vi "NAO_UTILIZAR_para_desenvolver.vi"() -> ()   [LabVIEW 2020]
uses:
  <vilib>/Rock Robotics/WPI/RobotDrive/WPI_RobotDriveArcadeDrive_Standard(NoSaturation).vi
  <vilib>/Rock Robotics/Network Tables/NT Read Number.vi
  Prog_Testes/GlobalVariables.vi
  <vilib>/Rock Robotics/Network Tables/NT Write Number.vi
  <vilib>/Rock Robotics/WPI/ThirdParty/Phoenix-LabVIEW/Motor Controller/Controls/CTRE_Phoenix_MotorControl_ControlMode.ctl
  <vilib>/functionblocks/FB Core/FB Core.xnode
  <vilib>/functionblocks/Control/PID/PID.vi
  <vilib>/functionblocks/NI_FunctionBlock Libraries.lvlib
  <vilib>/Rock Robotics/SystemInterfaces/DIO/FPGA_DIOPWMChannel.ctl
  <vilib>/Rock Robotics/WPI/PWM/WPI_PWMDeadband.ctl
  <vilib>/Rock Robotics/WPI/MotorControl/WPI_MotorControlType.ctl
  <vilib>/Rock Robotics/SystemInterfaces/DIO/FPGA_DIOChannel.ctl
  <vilib>/Rock Robotics/WPI/MotorControl/WPI_MotorControlDeviceRef.ctl
  <vilib>/Rock Robotics/WPI/RobotDrive/WPI_RobotDriveDevRef.ctl
panel:
  out "Distance":dbl
  in  "Stop_PID":bool=TRUE
  out "pidOut":dbl
  out "Stop_pid":bool=TRUE
  out "Stop_pid":bool=TRUE
  out "OUT_PUT 2":bool
  out "pwm_shot 2":dbl
  out "Disp_Valido 2":dbl
  out "Axes[1] 2":dbl
  out "Axes[2] 2":dbl
  out "Axes[3] 2":dbl
  in  "input cluster 2":T1
  out "L_Y 2":dbl
  out "L_X 2":dbl
  out "Motor Values  2":dbl[](array[numeric])
  out "RobotDriveDevRef 2":T2={"DevStatus"={"status"=FALSE, "code"=0, "source"=""}, "Motors[]"=[], "Square Inputs"=FALSE, "Max Output"=1.0}
  in  "x 2":dbl
  out "x+y 2":dbl
  in  "Mot_Min 2":dbl=0.35
  in  "Mot_Max 2":dbl=0.35
  out "Lime_Max 2":dbl=0.35
  out "Lime_Min 2":dbl=0.35
  out "Negar 2":bool
  out "output cluster 2":T8
  out "Multiplicação 6":dbl
  out "Buttons 15":bool
  out "Buttons 14":bool
  out "OUT 6":dbl
  out "Mutliple":dbl
  out "Buttons 13":bool
  out "Buttons 12":bool
  out "OUT 5":dbl
  out "Mutliple":dbl
  out "Buttons 11":bool
  out "Buttons 10":bool
  out "OUT 4":dbl
  out "OUT 3":dbl
  out "Buttons 9":bool
  out "Buttons 8":bool
  out "Multiplicação 3":dbl
  out "OUT_PUT":bool
  out "Disp_Valido":dbl
  out "pwm_shot":dbl
  out "Negar":bool
  out "Lime_Min":dbl=0.35
  out "Lime_Max":dbl=0.35
  in  "Mot_Max":dbl=0.35
  in  "Mot_Min":dbl=0.35
  out "x+y":dbl
  in  "x":dbl
  out "RobotDriveDevRef":T2={"DevStatus"={"status"=FALSE, "code"=0, "source"=""}, "Motors[]"=[], "Square Inputs"=FALSE, "Max Output"=1.0}
  out "Motor Values":dbl[](array[numeric])
  out "L_Y":dbl
  out "L_X":dbl
  in  "input cluster":T1
  out "Axes[3]":dbl
  out "Axes[2]":dbl
  out "Axes[1]":dbl
  out "output cluster":T8
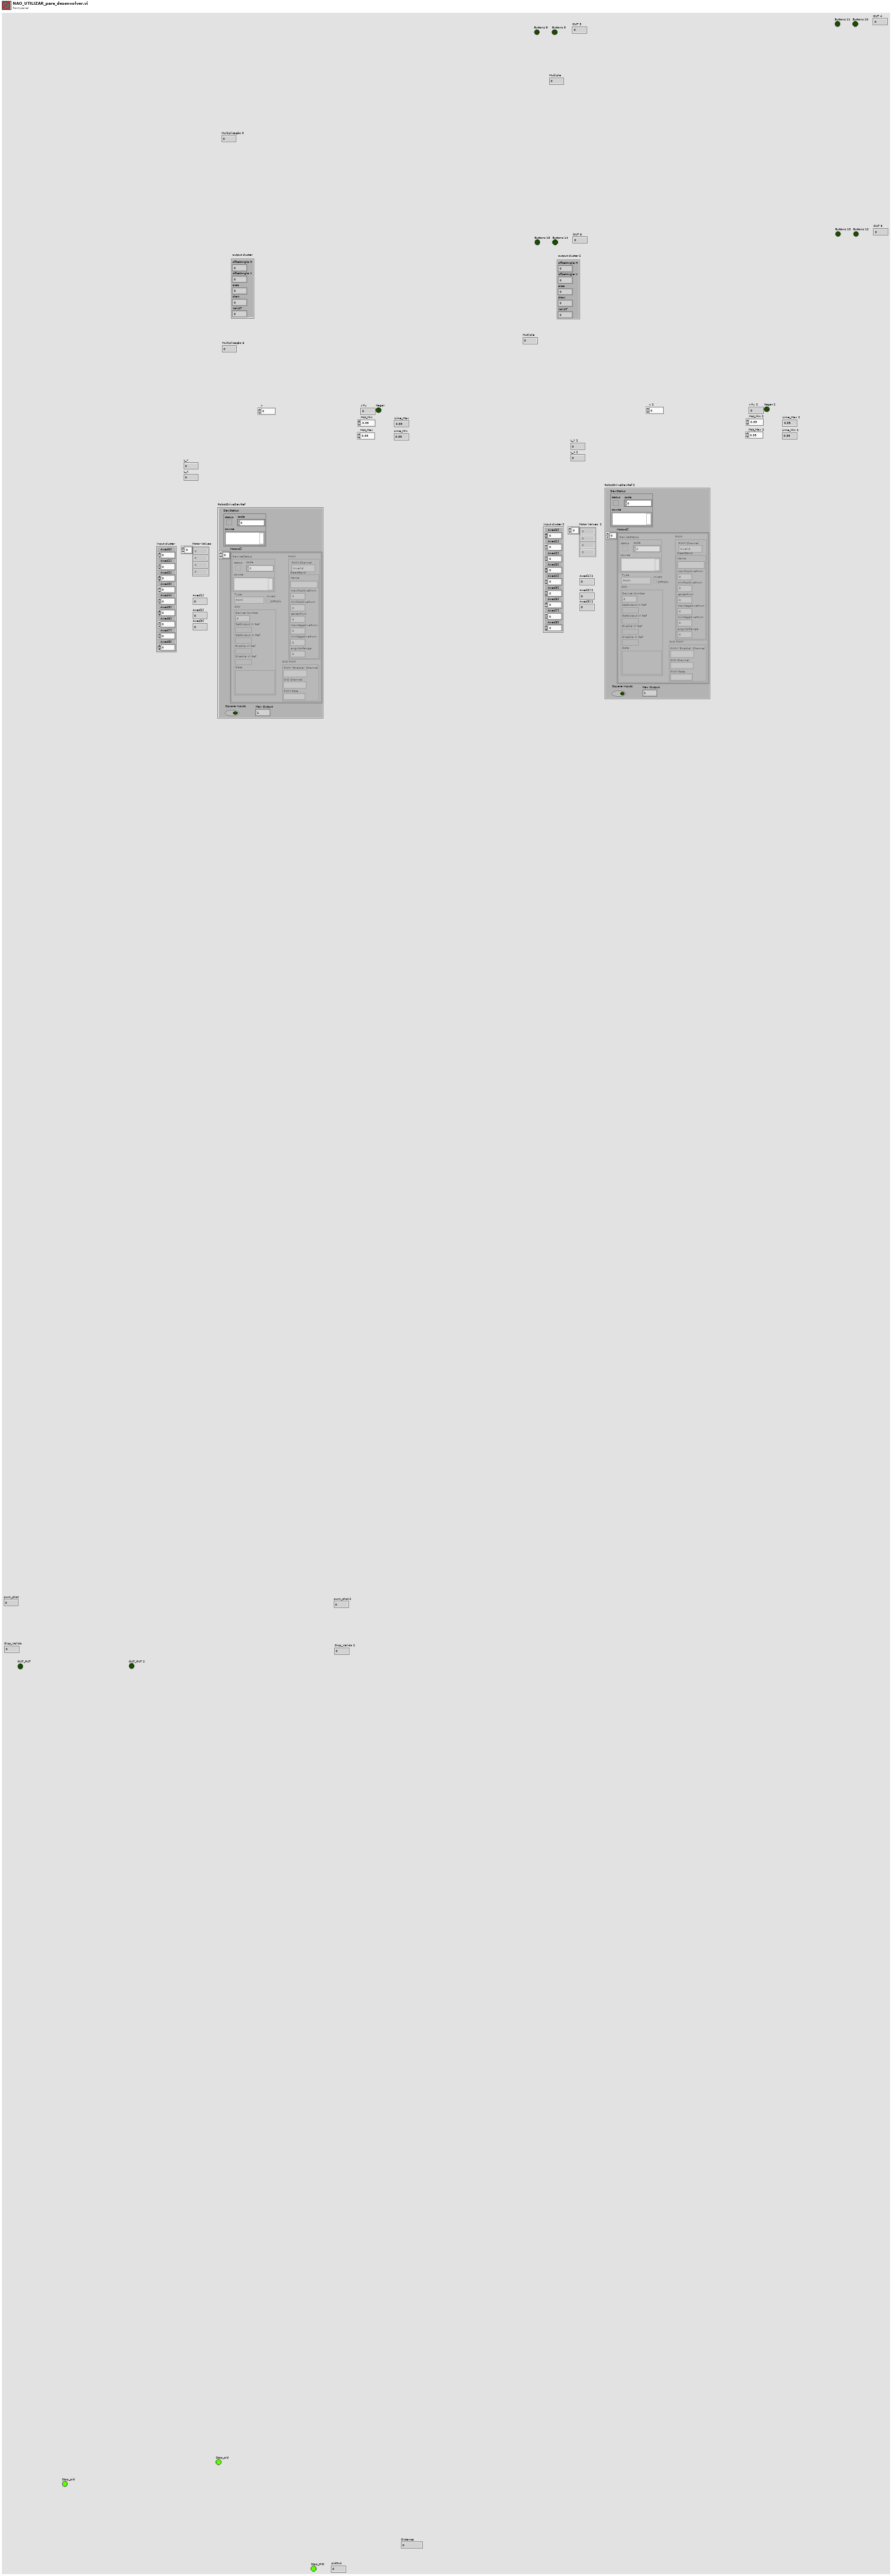
[diagram p1: front panel]
types:
  T1 = cluster{"Axes[0]":dbl, "Axes[1]":dbl, "Axes[2]":dbl, "Axes[3]":dbl, "Axes[4]":dbl, "Axes[5]":dbl, "Axes[6]":dbl, "Axes[7]":dbl, "Axes[8]":dbl}
  T2 = typedef "WPI_RobotDriveDevRef.ctl" = cluster{"DevStatus":errorcluster, "Motors[]":T3[], "Square Inputs":bool, "Max Output":dbl}
  T3 = typedef "WPI_MotorControlDeviceRef.ctl" = cluster{"DeviceStatus":errorcluster, "Type":T4, "PWM":cluster{"PWM Channel":T5, "DeadBand":T6}, "CAN":cluster{"Device Number":u8, "SetOutput VI Ref":variant, "GetOutput VI Ref":variant, "Enable VI Ref":variant, "Disable VI Ref":variant, "Data":variant}, "Invert":bool, "DIO PWM":cluster{"PWM \"Enable\" Channel":T5, "DIOChannel":T7, "PWM Rate":dbl}}
  T4 = typedef "WPI_MotorControlType.ctl" = enum16{"PWM", "CAN", "DIO PWM"}
  T5 = typedef "FPGA_DIOPWMChannel.ctl" = enum8{"PWM 0", "PWM 1", "PWM 2", "PWM 3", "PWM 4", "PWM 5", "PWM 6", "PWM 7", "PWM 8", "PWM 9", "PWM MXP 0", "PWM MXP 1", "PWM MXP 2", "PWM MXP 3", "PWM MXP 4", "PWM MXP 5", "PWM MXP 6", "PWM MXP 7", "PWM MXP 8", "PWM MXP 9", "Invalid"}
  T6 = typedef "WPI_PWMDeadband.ctl" = cluster{"Name":string, "maxPositivePwm":i32, "minPositivePwm":i32, "centerPwm":i32, "maxNegativePwm":i32, "minNegativePwm":i32, "angularRange":u16}
  T7 = typedef "FPGA_DIOChannel.ctl" = enum8{"DIO 0", "DIO 1", "DIO 2", "DIO 3", "DIO 4", "DIO 5", "DIO 6", "DIO 7", "DIO 8", "DIO 9", "DIO MXP 0", "DIO MXP 1", "DIO MXP 2", "DIO MXP 3", "DIO MXP 4", "DIO MXP 5", "DIO MXP 6", "DIO MXP 7", "DIO MXP 8", "DIO MXP 9", "DIO MXP 10", "DIO MXP 11", "DIO MXP 12", "DIO MXP 13", "DIO MXP 14", "DIO MXP 15", "SPI Port CS1", "SPI Port CS2", "SPI Port CS3", "SPI Port MISO", "SPI Port MOSI", "Invalid"}
  T8 = cluster{"offsetAngle H":dbl, "offsetAngle V":dbl, "area":dbl, "skew":dbl, "ValidT":dbl}
  T9 = typedef "CTRE_Phoenix_MotorControl_ControlMode.ctl" = u16
  T10 = cluster{"Buttons[0]":bool, "Buttons[1]":bool, "Buttons[2]":bool, "Buttons[3]":bool, "Buttons[4]":bool, "Buttons[5]":bool, "Buttons[6]":bool, "Buttons[7]":bool, "Buttons[8]":bool, "Buttons[9]":bool}
  T11 = typedef "WPI_JoystickDevRef.ctl" = cluster{"Device":T12}
  T12 = typedef "WPI_JoystickDeviceEnum.ctl" = enum16{"USB 0", "USB 1", "USB 2", "USB 3", "USB 4", "USB 5"}
  T13 = cluster{"Buttons[0]":bool, "Buttons[1]":bool, "Buttons[2]":bool, "Buttons[3]":bool, "Buttons[4]":bool, "Buttons[5]":bool, "Buttons[6]":bool, "Buttons[7]":bool, "Buttons[8]":bool}
  T14 = cluster{"POVs[0]":i16, "POVs[1]":i16, "POVs[2]":i16, "POVs[3]":i16, "POVs[4]":i16, "POVs[5]":i16, "POVs[6]":i16, "POVs[7]":i16}
  T15 = typedef "WPI_EncoderDevRef.ctl" = cluster{"DevStatus":errorcluster, "EncoderIndex":T16, "CounterIndex":T17, "DistancePerCount":dbl, "Decoding Type":T18}
  T16 = typedef "FPGA_EncoderIdx.ctl" = enum8{"Enc 0", "Enc 1", "Enc 2", "Enc 3", "Enc 4", "Enc 5", "Enc 6", "Enc 7", "Invalid"}
  T17 = typedef "FPGA_CounterCtrSystemIndex.ctl" = enum8{"Ctr 0", "Ctr 1", "Ctr 2", "Ctr 3", "Ctr 4", "Ctr 5", "Ctr 6", "Ctr 7", "Invalid"}
  T18 = typedef "WPI_EncoderType.ctl" = enum16{"1x", "2x", "4x"}
  T19 = cluster{"Axes[0]":dbl, "Axes[1]":dbl, "Axes[2]":dbl, "Axes[3]":dbl}
  T20 = cluster{"Axes[0]":dbl, "Axes[1]":dbl, "Axes[2]":dbl, "Axes[3]":dbl, "Axes[4]":dbl, "Axes[5]":dbl, "Axes[6]":dbl, "Axes[7]":dbl}
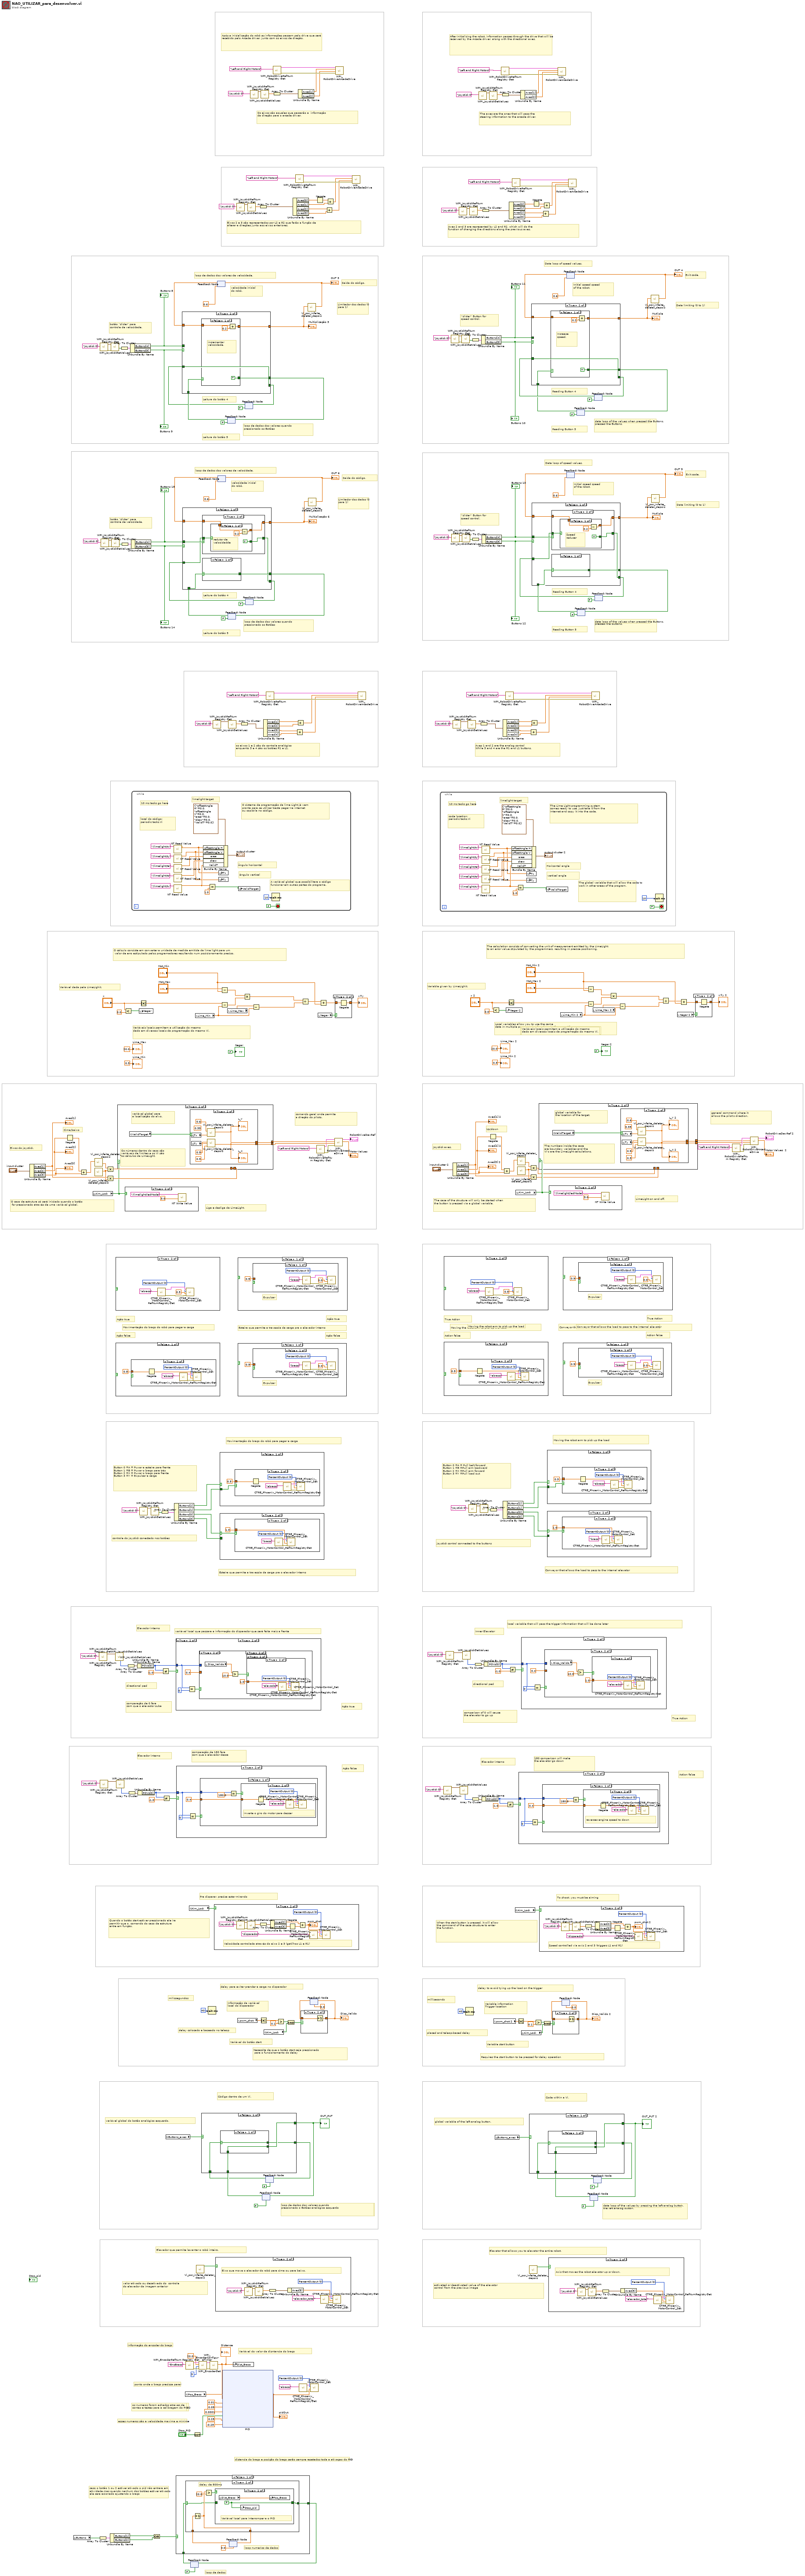
[diagram p0: block diagram]
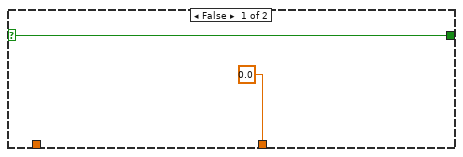
[diagram p2: hidden frame]
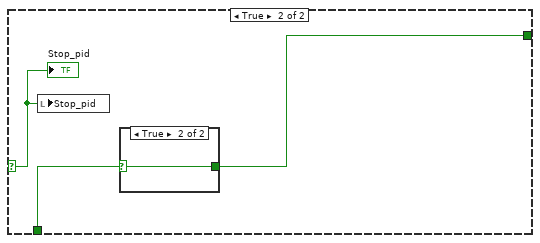
[diagram p4: hidden frame]
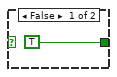
[diagram p5: hidden frame]
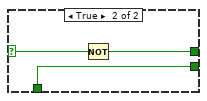
[diagram p6: hidden frame]
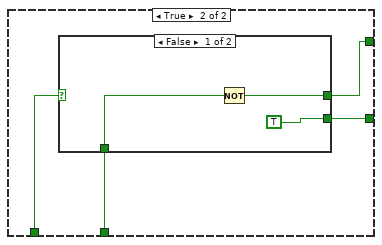
[diagram p7: hidden frame]
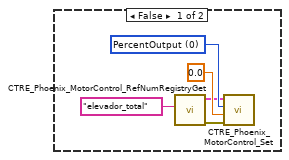
[diagram p9: hidden frame]
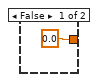
[diagram p10: hidden frame]
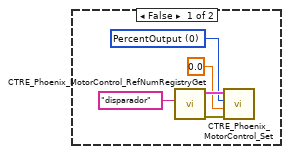
[diagram p11: hidden frame]
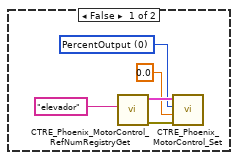
[diagram p12: hidden frame]
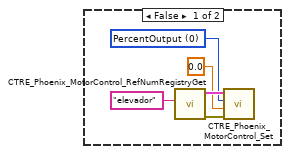
[diagram p13: hidden frame]
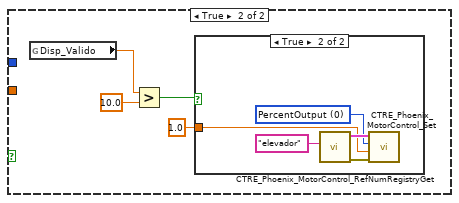
[diagram p14: hidden frame]
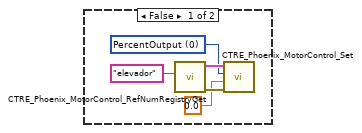
[diagram p15: hidden frame]
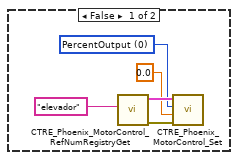
[diagram p16: hidden frame]
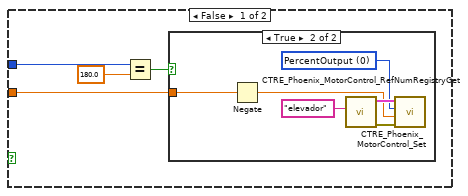
[diagram p17: hidden frame]
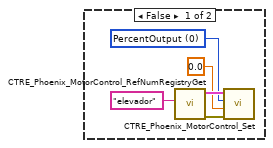
[diagram p18: hidden frame]
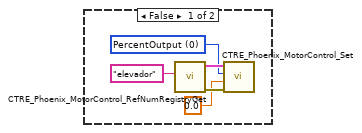
[diagram p19: hidden frame]
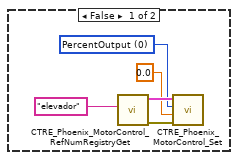
[diagram p20: hidden frame]
diagram:
  w20 = T9 0 items=["PercentOutput"=0, "Position"=1, "Velocity"=2, "Current"=3, "Follower"=5, "MotionProfile"=6, "MotionMagic"=7, "MotionProfileArc"=10, "Disabled"=15] ("Control Mode")
  # "distancia do braço e posição do breço serão sempre resetados toda a ativaçao do PID"
  # "distancia do braço e posição do breço serão sempre resetados toda a ativaçao do PID"
  # "caso o botão 1 ou 2 estiver ativado o pid não entrara em \natividade,mas quando nenhum dos botões estiver ativado \nele sera acionado ajustando o braço"
  # "loop de dados"
  # "esses numeros são a velocidade maxima e minima"
  # "esses numeros são a velocidade maxima e minima"
  # "os numeros forom achados atravez de \ncalculos e testes para a calibragem do PID"
  # "os numeros forom achados atravez de \ncontas e testes para a calibragem do PID"
  # "os numeros forom achados atravez de \ncontas e testes para a calibragem do PID"
  # "ponto onde o braço precissa parar"
  # "Variável do valor da disntancia do braço"
  # "informação do encoder do braço"
  # "activated or deactivated value of the elevator \ncontrol from the previous image"
  # "Code within a Vi."
  # "data loop of the values by pressed \nthe left analog button."
  # "data loop of the values by pressing the left analog button."
  # "global variable of the left analog button."
  # "Elevator that allows you to elevator the entire robot."
  # "To shoot, you must be aiming"
  # "Variable start button"
  # "Requires the start button to be pressed for delay operation"
  # "Variable information \nTrigger location"
  # "milliseconds"
  # "placed and teleop-based delay"
  # "When the start button is pressed, it will allow\nthe command of the case structure to enter \nthe function."
  # "delay to avoid tying up the load on the trigger"
  # "Action false"
  # "180 comparison will make \nthe elevator go down"
  # "Elevador interno"
  # "True Action"
  # "comparison of 0 will cause \nthe elevator to go up"
  # "local variable that will pass the trigger information that will be done later"
  # "directional ped"
  # "Inner Elevator"
  # "Ação true"
  # "comparação de 0 fara \ncom que o elevador suba"
  # "variável local que passara a informação do disparador que será feita mais a frente"
  # "directional ped"
  # "Elevador interno"
  # "joystick control connected to the buttons"
  # "Conveyor that allows the load to pass to the internal elevator"
  # "Moving the robot arm to pick up the load"
  # "Button 0 =A = Pull belt forward  \nButton 1 =B =Pull arm backward \nButton 2 =X =Pull arm forward  \nButton 3 =Y =Pull load out"
  # "Moving the robot arm to pick up the load"
  # "Conveyor that allows the load to pass to the internal elevator"
  # "Action false"
  # "True Action"
  # "True Action"
  # "Action false"
  # "Conveyor that allows the load to pass to the internal elevator"
  # "Moving the robot arm to pick up the load"
  # "general command where it \nallows the pilot's direction."
  # "The case of the structure will only be started when\nthe button is pressed via a global variable."
  # "LimeLight on and off."
  # "Joystick axes."
  # "Up/down"
  # "Local variables allow you to use the same \ndata in multiple programming locations in the same Vi."
  # "Variáveis locais permitem a utilização do mesmo \ndado em diversos locais da programação do mesmo Vi."
  # "Variáveis locais permitem a utilização do mesmo \ndado em diversos locais da programação do mesmo Vi."
  # "Variable given by LimeLighit."
  # "The calculation consists of converting the unit of measurement emitted by the LimeLight \nto an error value stipulated by the programmers, resulting in precise positioning."
  # "Axes 1 and 2 are the analog control \nWhile 3 and 4 are the R1 and L1 buttons."
  # "Data loop of the values when \npressed the Buttons."
  # "data loop of the values when pressed the Buttons."
  # "Data loop of speed values."
  # "''slider'' Button for \nspeed control."
  # "Initial speed speed \nof the robot."
  # "Data limiting (0 to 1)"
  # "Exit code."
  # "Reading Button 5"
  # "Reading Button 4"
  # "loop de dados dos valores quando \npressionado os Botões."
  # "loop de dados dos valores quando \npressionado os Botões"
  # "loop de dados dos valores de velocidade."
  # "botão “slider” para \ncontrole de velocidade."
  # "velocidade inicial \ndo robô."
  # "Limitador dos dados (0 para 1)"
  # "Saída do código."
  # "Leitura do botão 5"
  # "Leitura do botão 4"
  # "Data loop of the values when \npressed the Buttons."
  # "data loop of the values when pressed the Buttons."
  # "Data loop of speed values."
  # "''slider'' Button for \nspeed control."
  # "Initial speed speed \nof the robot."
  # "Data limiting (0 to 1)"
  # "Exit code."
  # "Reading Button 5"
  # "Reading Button 4"
  # "Axes 2 and 3 are represented by L2 and R2, which will do the\nfunction of changing the directions along the previous axes."
  # "The axes are the ones that will pass the \nsteering information to the arcade driver."
  # "After initializing the robot, information passes through the drive that will be received by the Arcade driver, along with the directional axes."
  # "valor ativado ou desativado do  controle \ndo elevador da imagem anterior"
  # "Código dentro de um Vi."
  # "Variáveis locais permitem a utilização do mesmo \ndado em diversos locais da programação do mesmo Vi."
  # "Variáveis locais permitem a utilização do mesmo \ndado em diversos locais da programação do mesmo Vi."
  # "loop de dados dos valores quando \npressionado os Botões."
  # "loop de dados dos valores quando \npressionado os Botões"
  # "loop de dados dos valores de velocidade."
  # "botão “slider” para \ncontrole de velocidade."
  # "velocidade inicial \ndo robô."
  # "Limitador dos dados (0 para 1)"
  # "Saída do código."
  # "Leitura do botão 5"
  # "Leitura do botão 4"
  # "loop de dados dos valores quando \npressionado o Botões analógico esquerdo."
  # "loop de dados dos valores quando \npressionado o Botões analógico esquerdo"
  # "variável global do botão analógico esquerdo."
  # "Elevador que permite levantar o robô inteiro."
  # "Variável do botão start"
  # "Necessita de que o botão start seja pressionado\n para o funcionamento do delay"
  # "Informação da variável \nlocal do disparador"
  # "milissegundos"
  # "delay colocado e baseado no teleop"
  # "Quando o botão start estiver pressionado ele ira \npermitir que o  comando do caso de estrutura \nentre em função."
  # "delay para evitar prender a carga no disparador"
  # "Pra disparar, precisa estar mirando"
  # "Ação false"
  # "Ação true"
  # "comparação de 0 fara \ncom que o elevador suba"
  # "comparação de 180 fara \ncom que o elevador dessa"
  # "variável local que passara a informação do disparador que será feita mais a frente"
  # "directional ped"
  # "Elevador interno"
  # "controle do joystick conectado nos botões"
  # "Esteira que permite a travessia da carga pra o elevador interno"
  # "Movimentação do braço do robô para pegar a carga"
  # "Button 0 =A = Puxar a esteira para frente  \nButton 1 =B = Puxar o braço para trás \nButton 2 =X = Puxar o braço para frente  \nButton 3 =Y = Expulsar a carga"
  # "Movimentação do braço do robô para pegar a carga"
  # "Esteira que permite a travessia da carga pra o elevador interno"
  # "Ação false"
  # "Ação true"
  # "Ação true"
  # "Ação false"
  # "Esteira que permite a travessia da carga pra o elevador interno"
  # "Movimentação do braço do robô para pegar a carga"
  # "Elevador interno"
  # "comando geral onde permite \na direção do piloto."
  # "O caso de estrutura só será iniciado quando o botão\n for pressionado através de uma variável global."
  # "Liga e desliga da LimeLight."
  # "os eixos 1 e 2 são do controle analógico \nenquanto 3 e 4 são os botões R1 e L1."
  # "Eixos do joystick."
  # "Variáveis locais permitem a utilização do mesmo \ndado em diversos locais da programação do mesmo Vi."
  # "Variável dada pela LimeLighit."
  # "O cálculo consiste em converter a unidade de medida emitida da lime light para um\n valor de erro estipulado pelos programadores resultando num posicionamento preciso."
  # "Cima/baixo"
  # "Eixos 2 e 3 são representados por L2 e R2 que farão a função de  \nalterar a direções junto aos eixos anteriores."
  # "Os eixos são aqueles que passarão a  informação\nda direção para o arcade driver."
  # "Após a inicialização do robô as informações passam pelo drive que será recebido pelo Arcade driver, junto com os eixos de direção."
  n1 = Unbundle By Name("input cluster") -> ("Axes[1]"=w309:dbl, "Axes[2]"=w308:dbl, "Axes[3]"=w295:dbl)
  "Axes[1]" <- w309
  "Axes[2]" <- w308
  "Axes[3]" <- w295
  n2 = Negate(x=w308) -> (-x=w307:dbl)
  n3 = global read "GlobalVariables.vi" "Buttons"() -> (w3:bool[])
  n4 = Add(x=w307, y=w295) -> (x+y=w274:dbl)
  n5 = global read "GlobalVariables.vi" "Aim_Lock"() -> (w296:bool)
  n6 = call "Vi_por_infeite_deletar_depois.vi"("Numeric"=w274) -> ("Numeric 4"=w275:dbl)  [unwired: 8 in, 2 out]
  n7 = call "Vi_por_infeite_deletar_depois.vi"() -> ("Numeric 3"=w273:dbl)  [unwired: 9 in, 2 out]
  n8 = Array To Cluster(array=w3) -> (cluster=w4:T10)
  n9 = call <vilib>:"WPI_JoystickRefNum Registry Get.vi"("refnum name"="Joystick 0") -> ("JoystickDevRef"=w63:T11)  [unwired: 1 in, 9 out]
  n10 = call <vilib>:"WPI_JoystickRefNum Registry Get.vi"("refnum name"="Joystick 0") -> ("JoystickDevRef"=w259:T11)  [unwired: 1 in, 9 out]
  n11 = call <vilib>:"WPI_JoystickRefNum Registry Get.vi"("refnum name"="Joystick 0") -> ("JoystickDevRef"=w238:T11)  [unwired: 1 in, 9 out]
  n12 = call <vilib>:"WPI_JoystickRefNum Registry Get.vi"("refnum name"="Joystick 0") -> ("error out"=w210:errorcluster, "JoystickDevRef"=w209:T11)  [unwired: 1 in, 8 out]
  n13 = call <vilib>:"WPI_JoystickRefNum Registry Get.vi"("refnum name"="Joystick 0") -> ("error out"=w137:errorcluster, "JoystickDevRef"=w138:T11)  [unwired: 1 in, 8 out]
  n14 = Multiply(x=w275, y=w273) -> (x*y=w304:dbl)
  n15 = Multiply(x=w309, y=w273) -> (x*y=w305:dbl)
  n16 = Unbundle By Name(w4) -> ("Buttons[1]"=w2:bool, "Buttons[2]"=w1:bool)
  n17 = call <vilib>:"WPI_JoystickGetValues.vi"("error in (no error)"=w210, "JoystickDevRef"=w209) -> ("Buttons"=w207:bool[])  [unwired: 5 in, 4 out]
  n18 = call <vilib>:"WPI_JoystickGetValues.vi"("error in (no error)"=w137, "JoystickDevRef"=w138) -> ("Buttons"=w140:bool[])  [unwired: 5 in, 4 out]
  n19 = call <vilib>:"WPI_JoystickGetValues.vi"("JoystickDevRef"=w63) -> ("POVs"=w67:i16[])  [unwired: 6 in, 4 out]
  n20 = call <vilib>:"WPI_JoystickGetValues.vi"("JoystickDevRef"=w259) -> ("POVs"=w255:i16[])  [unwired: 6 in, 4 out]
  n21 = case shown="True" {
    selector: _ -> [_ _]
    frame False {
      n22 = case shown="True" {
        selector: _ -> [_ _]
        tunnel: 0.5 ("Output") -> [_ w340]
        frame False {
          w335 = T9 0 items=["PercentOutput"=0, "Position"=1, "Velocity"=2, "Current"=3, "Follower"=5, "MotionProfile"=6, "MotionMagic"=7, "MotionProfileArc"=10, "Disabled"=15] ("Control Mode")
          n23 = call <vilib>:"CTRE_Phoenix_MotorControl_RefNumRegistryGet.vi"("refnum name"="abraco") -> ("error out"=w337:errorcluster, "PhoenixMotorControlDevRef"=w338:T3)  [unwired: 9 in]
          n24 = call <vilib>:"CTRE_Phoenix_MotorControl_Set.vi"("error in (no error)"=w337, "Output"=0.0, "Control Mode"=w335, "PhoenixMotorControlDevRef"=w338) -> ()  [unwired: 6 in, 2 out]
        }
        frame True {
          w341 = T9 0 items=["PercentOutput"=0, "Position"=1, "Velocity"=2, "Current"=3, "Follower"=5, "MotionProfile"=6, "MotionMagic"=7, "MotionProfileArc"=10, "Disabled"=15] ("Control Mode")
          n25 = Negate(x=w340) -> (-x=w339:dbl)
          n26 = call <vilib>:"CTRE_Phoenix_MotorControl_RefNumRegistryGet.vi"("refnum name"="abraco") -> ("error out"=w343:errorcluster, "PhoenixMotorControlDevRef"=w342:T3)  [unwired: 9 in]
          n27 = call <vilib>:"CTRE_Phoenix_MotorControl_Set.vi"("error in (no error)"=w343, "Output"=w339, "Control Mode"=w341, "PhoenixMotorControlDevRef"=w342) -> ()  [unwired: 6 in, 2 out]
        }
      }
    }
    frame True {
      w345 = T9 0 items=["PercentOutput"=0, "Position"=1, "Velocity"=2, "Current"=3, "Follower"=5, "MotionProfile"=6, "MotionMagic"=7, "MotionProfileArc"=10, "Disabled"=15] ("Control Mode")
      n28 = call <vilib>:"CTRE_Phoenix_MotorControl_RefNumRegistryGet.vi"("refnum name"="abraco") -> ("error out"=w347:errorcluster, "PhoenixMotorControlDevRef"=w348:T3)  [unwired: 9 in]
      n29 = call <vilib>:"CTRE_Phoenix_MotorControl_Set.vi"("error in (no error)"=w347, "Output"=0.5, "Control Mode"=w345, "PhoenixMotorControlDevRef"=w348) -> ()  [unwired: 6 in, 2 out]
    }
  }
  n30 = case shown="False" {
    selector: _ -> [_ _]
    frame False {
      n31 = case shown="True" {
        selector: _ -> [_ _]
        tunnel: 0.5 ("Output") -> [_ w357]
        frame False {
          w352 = T9 0 items=["PercentOutput"=0, "Position"=1, "Velocity"=2, "Current"=3, "Follower"=5, "MotionProfile"=6, "MotionMagic"=7, "MotionProfileArc"=10, "Disabled"=15] ("Control Mode")
          n32 = call <vilib>:"CTRE_Phoenix_MotorControl_RefNumRegistryGet.vi"("refnum name"="abraco") -> ("error out"=w354:errorcluster, "PhoenixMotorControlDevRef"=w355:T3)  [unwired: 9 in]
          n33 = call <vilib>:"CTRE_Phoenix_MotorControl_Set.vi"("error in (no error)"=w354, "Output"=0.0, "Control Mode"=w352, "PhoenixMotorControlDevRef"=w355) -> ()  [unwired: 6 in, 2 out]
        }
        frame True {
          w358 = T9 0 items=["PercentOutput"=0, "Position"=1, "Velocity"=2, "Current"=3, "Follower"=5, "MotionProfile"=6, "MotionMagic"=7, "MotionProfileArc"=10, "Disabled"=15] ("Control Mode")
          n34 = Negate(x=w357) -> (-x=w356:dbl)
          n35 = call <vilib>:"CTRE_Phoenix_MotorControl_RefNumRegistryGet.vi"("refnum name"="abraco") -> ("error out"=w360:errorcluster, "PhoenixMotorControlDevRef"=w359:T3)  [unwired: 9 in]
          n36 = call <vilib>:"CTRE_Phoenix_MotorControl_Set.vi"("error in (no error)"=w360, "Output"=w356, "Control Mode"=w358, "PhoenixMotorControlDevRef"=w359) -> ()  [unwired: 6 in, 2 out]
        }
      }
    }
    frame True {
      w362 = T9 0 items=["PercentOutput"=0, "Position"=1, "Velocity"=2, "Current"=3, "Follower"=5, "MotionProfile"=6, "MotionMagic"=7, "MotionProfileArc"=10, "Disabled"=15] ("Control Mode")
      n37 = call <vilib>:"CTRE_Phoenix_MotorControl_RefNumRegistryGet.vi"("refnum name"="abraco") -> ("error out"=w364:errorcluster, "PhoenixMotorControlDevRef"=w365:T3)  [unwired: 9 in]
      n38 = call <vilib>:"CTRE_Phoenix_MotorControl_Set.vi"("error in (no error)"=w364, "Output"=0.5, "Control Mode"=w362, "PhoenixMotorControlDevRef"=w365) -> ()  [unwired: 6 in, 2 out]
    }
  }
  n39 = call <vilib>:"WPI_JoystickGetValues.vi"("JoystickDevRef"=w238) -> ("POVs"=w242:i16[])  [unwired: 6 in, 4 out]
  n40 = case shown="True" w296 {
    tunnel: w305 -> [w368 _]
    tunnel: w304 -> [w367 _]
    tunnel: [w368 w370] -> w303
    tunnel: [w367 w371] -> w302
    frame False {
    }
    frame True {
      # "Os números dentro do caso são \nvariáveis de limites e os Vi são \nos cálculos da LimeLight."
      # "variável global para \na localização do alvo."
      n41 = global read "GlobalVariables.vi" "ValidTarget"() -> (w369:bool)
      n42 = case shown="True" w369 {
        tunnel: [0.0 ("x+y") w378] -> w371
        tunnel: [0.0 ("x+y") w374] -> w370
        frame False {
        }
        frame True {
          (unwired) 0.35
          n43 = global read "GlobalVariables.vi" "Tx"() -> (w379:dbl)
          n44 = global read "GlobalVariables.vi" "Ty"() -> (w376:dbl)
          n45 = call "Vi_por_infeite_deletar_depois.vi"("Numeric 2"=w379, "Numeric"=0.6) -> ("Numeric 3"=w378:dbl)  [unwired: 7 in, 2 out]
          "L_Y" <- w378
          n46 = call "Vi_por_infeite_deletar_depois.vi"("Numeric 5"=0.3, "Numeric 2"=w376, "Numeric"=0.9) -> ("Numeric 4"=w374:dbl)  [unwired: 6 in, 2 out]
          "L_X" <- w374
        }
      }
    }
  }
  n47 = Array To Cluster(array=w207) -> (cluster=w219:T13)
  n48 = Array To Cluster(array=w140) -> (cluster=w128:T13)
  n49 = Less?(x="x", y=0.0) -> (x < y?=w283:bool)
  n50 = case shown="True" w296 {
    frame False {
      n51 = call-poly <vilib>:"NT Write Value.vi"("Numeric"=1.0, "Name"="/limelight/ledMode") -> ()  [unwired: 9 in, 1 out]
    }
    frame True {
      n52 = call-poly <vilib>:"NT Write Value.vi"("Numeric"=3.0, "Name"="/limelight/ledMode") -> ()  [unwired: 9 in, 1 out]
    }
  }
  n53 = Array To Cluster(array=w67) -> (cluster=w68:T14)
  n54 = Array To Cluster(array=w255) -> (cluster=w254:T14)
  n55 = Array To Cluster(array=w242) -> (cluster=w243:T14)
  n56 = Unbundle By Name(w219) -> ("Buttons[4]"=w218:bool, "Buttons[5]"=w217:bool)
  "Buttons 8" <- w218
  "Buttons 9" <- w217
  n57 = Unbundle By Name(w128) -> ("Buttons[4]"=w129:bool, "Buttons[5]"=w130:bool)
  "Buttons 15" <- w129
  "Buttons 14" <- w130
  n58 = while {
    stop <- FALSE stop-if-true
    # "local do código: \nperiodic tasks.Vi"
    # "A variável global que possibilitara o código  \nfuncionar em outras partes do programa."
    # "O sistema de programação da lime Light já vem  \npronta para se utilizar basta pegar na internet  \nou copiá-la no código."
    # "ângulo vertical"
    # "Ângulo horizontal"
    # "limelight target"
    # "10 ms tasks go here"
    n59 = call-poly <vilib>:"NT Read Value.vi"("Name"="/limelight/tx") -> ("Numeric"=w387:dbl)  [unwired: 9 in, 1 out]
    n60 = call-poly <vilib>:"NT Read Value.vi"("Name"="/limelight/ty") -> ("Numeric"=w386:dbl)  [unwired: 9 in, 1 out]
    n61 = call-poly <vilib>:"NT Read Value.vi"("Name"="/limelight/ta") -> ("Numeric"=w394:dbl)  [unwired: 9 in, 1 out]
    n62 = call-poly <vilib>:"NT Read Value.vi"("Name"="/limelight/ts") -> ("Numeric"=w395:dbl)  [unwired: 9 in, 1 out]
    n63 = call-poly <vilib>:"NT Read Value.vi"("Name"="/limelight/tv") -> ("Numeric"=w388:dbl)  [unwired: 9 in, 1 out]
    n64 = Bundle By Name(cluster=T8 {"offsetAngle H"=0.0, "offsetAngle V"=0.0, "area"=0.0, "skew"=0.0, "ValidT"=0.0} ("input cluster"), "offsetAngle H"=w387, "offsetAngle V"=w386, "area"=w394, "skew"=w395, "ValidT"=w388) -> (→"output cluster":T8)
    n65 = Equal?(x=w388, y=1.0) -> (x = y?=w385:bool)
    n66 = global write "GlobalVariables.vi" "Tx"(w387) -> ()
    n67 = global write "GlobalVariables.vi" "Ty"(w386) -> ()
    n68 = global write "GlobalVariables.vi" "ValidTarget"(w385) -> ()
    n69 = Wait (ms)(milliseconds to wait=u32 10) -> ()  [unwired: 1 out]
  }
  n70 = Unbundle By Name(w68) -> ("POVs[0]"=w69:i16)
  n71 = Unbundle By Name(w254) -> ("POVs[0]"=w253:i16)
  n72 = Unbundle By Name(w243) -> ("POVs[0]"=w244:i16)
  n73 = local write "Negar"(w283) -> ()
  n74 = Absolute Value(x="x") -> (abs(x)=w281:dbl)
  n75 = call <vilib>:"WPI_JoystickRefNum Registry Get.vi"("refnum name"="Joystick 0") -> ("JoystickDevRef"=w251:T11)  [unwired: 1 in, 9 out]
  n76 = call <vilib>:"WPI_JoystickGetValues.vi"("JoystickDevRef"=w251) -> ("Buttons"=w250:bool[])  [unwired: 6 in, 4 out]
  n77 = Or(x=w2, y=w1) -> (x .or. y?=w26:bool)
  n78 = Array To Cluster(array=w250) -> (cluster=w249:T10)
  n79 = Not Equal?(x=w69, y=-1.0) -> (x != y?=w66:bool)
  n80 = Not Equal?(x=w253, y=-1.0) -> (x != y?=w256:bool)
  n81 = Not Equal?(x=w244, y=-1.0) -> (x != y?=w241:bool)
  n82 = global read "GlobalVariables.vi" "Buttons_axes"() -> (w202:bool)
  n83 = Unbundle By Name(w249) -> ("Buttons[2]"=w245:bool, "Buttons[1]"=w246:bool, "Buttons[0]"=w248:bool, "Buttons[3]"=w247:bool)
  n84 = case shown="True" w66 {
    tunnel: w69 -> [_ w407]
    frame False {
      w402 = T9 0 items=["PercentOutput"=0, "Position"=1, "Velocity"=2, "Current"=3, "Follower"=5, "MotionProfile"=6, "MotionMagic"=7, "MotionProfileArc"=10, "Disabled"=15] ("Control Mode")
      n85 = call <vilib>:"CTRE_Phoenix_MotorControl_RefNumRegistryGet.vi"("refnum name"="elevador") -> ("error out"=w404:errorcluster, "PhoenixMotorControlDevRef"=w405:T3)  [unwired: 9 in]
      n86 = call <vilib>:"CTRE_Phoenix_MotorControl_Set.vi"("error in (no error)"=w404, "Output"=0.0, "Control Mode"=w402, "PhoenixMotorControlDevRef"=w405) -> ()  [unwired: 6 in, 2 out]
    }
    frame True {
      n87 = Equal?(x=w407, y=i16 0) -> (x = y?=w408:bool)
      n88 = case shown="True" w408 {
        tunnel: w407 -> [w411 _]
        tunnel: 0.4 ("Output") -> [w410 _]
        frame False {
          n89 = Equal?(x=w411, y=180.0) -> (x = y?=w413:bool)
          n90 = case shown="True" w413 {
            tunnel: w410 -> [_ w419]
            frame False {
              w416 = T9 0 items=["PercentOutput"=0, "Position"=1, "Velocity"=2, "Current"=3, "Follower"=5, "MotionProfile"=6, "MotionMagic"=7, "MotionProfileArc"=10, "Disabled"=15] ("Control Mode")
              n91 = call <vilib>:"CTRE_Phoenix_MotorControl_RefNumRegistryGet.vi"("refnum name"="elevador") -> ("error out"=w417:errorcluster, "PhoenixMotorControlDevRef"=w418:T3)  [unwired: 9 in]
              n92 = call <vilib>:"CTRE_Phoenix_MotorControl_Set.vi"("error in (no error)"=w417, "Output"=0.0, "Control Mode"=w416, "PhoenixMotorControlDevRef"=w418) -> ()  [unwired: 6 in, 2 out]
            }
            frame True {
              w422 = T9 0 items=["PercentOutput"=0, "Position"=1, "Velocity"=2, "Current"=3, "Follower"=5, "MotionProfile"=6, "MotionMagic"=7, "MotionProfileArc"=10, "Disabled"=15] ("Control Mode")
              n93 = Negate(x=w419) -> (-x=w420:dbl)
              n94 = call <vilib>:"CTRE_Phoenix_MotorControl_RefNumRegistryGet.vi"("refnum name"="elevador") -> ("error out"=w423:errorcluster, "PhoenixMotorControlDevRef"=w424:T3)  [unwired: 9 in]
              n95 = call <vilib>:"CTRE_Phoenix_MotorControl_Set.vi"("error in (no error)"=w423, "Output"=w420, "Control Mode"=w422, "PhoenixMotorControlDevRef"=w424) -> ()  [unwired: 6 in, 2 out]
            }
          }
        }
        frame True {
          n96 = local read "Disp_Valido"() -> (w427:dbl)
          n97 = Greater?(x=w427, y=10.0) -> (0:w428:bool)
          n98 = case shown="True" w428 {
            tunnel: 1.0 ("Output") -> [_ w434]
            frame False {
              w431 = T9 0 items=["PercentOutput"=0, "Position"=1, "Velocity"=2, "Current"=3, "Follower"=5, "MotionProfile"=6, "MotionMagic"=7, "MotionProfileArc"=10, "Disabled"=15] ("Control Mode")
              n99 = call <vilib>:"CTRE_Phoenix_MotorControl_RefNumRegistryGet.vi"("refnum name"="elevador") -> ("error out"=w432:errorcluster, "PhoenixMotorControlDevRef"=w433:T3)  [unwired: 9 in]
              n100 = call <vilib>:"CTRE_Phoenix_MotorControl_Set.vi"("error in (no error)"=w432, "Output"=0.0, "Control Mode"=w431, "PhoenixMotorControlDevRef"=w433) -> ()  [unwired: 6 in, 2 out]
            }
            frame True {
              w436 = T9 0 items=["PercentOutput"=0, "Position"=1, "Velocity"=2, "Current"=3, "Follower"=5, "MotionProfile"=6, "MotionMagic"=7, "MotionProfileArc"=10, "Disabled"=15] ("Control Mode")
              n101 = call <vilib>:"CTRE_Phoenix_MotorControl_RefNumRegistryGet.vi"("refnum name"="elevador") -> ("error out"=w437:errorcluster, "PhoenixMotorControlDevRef"=w438:T3)  [unwired: 9 in]
              n102 = call <vilib>:"CTRE_Phoenix_MotorControl_Set.vi"("error in (no error)"=w437, "Output"=w434, "Control Mode"=w436, "PhoenixMotorControlDevRef"=w438) -> ()  [unwired: 6 in, 2 out]
            }
          }
        }
      }
    }
  }
  n103 = case shown="True" w256 {
    tunnel: w253 -> [_ w445]
    frame False {
      w440 = T9 0 items=["PercentOutput"=0, "Position"=1, "Velocity"=2, "Current"=3, "Follower"=5, "MotionProfile"=6, "MotionMagic"=7, "MotionProfileArc"=10, "Disabled"=15] ("Control Mode")
      n104 = call <vilib>:"CTRE_Phoenix_MotorControl_RefNumRegistryGet.vi"("refnum name"="elevador") -> ("error out"=w442:errorcluster, "PhoenixMotorControlDevRef"=w443:T3)  [unwired: 9 in]
      n105 = call <vilib>:"CTRE_Phoenix_MotorControl_Set.vi"("error in (no error)"=w442, "Output"=0.0, "Control Mode"=w440, "PhoenixMotorControlDevRef"=w443) -> ()  [unwired: 6 in, 2 out]
    }
    frame True {
      n106 = Equal?(x=w445, y=i16 0) -> (x = y?=w446:bool)
      n107 = case shown="True" w446 {
        tunnel: w445 -> [w449 _]
        tunnel: 0.4 ("Output") -> [w448 _]
        frame False {
          n108 = Equal?(x=w449, y=180.0) -> (x = y?=w451:bool)
          n109 = case shown="True" w451 {
            tunnel: w448 -> [_ w457]
            frame False {
              w454 = T9 0 items=["PercentOutput"=0, "Position"=1, "Velocity"=2, "Current"=3, "Follower"=5, "MotionProfile"=6, "MotionMagic"=7, "MotionProfileArc"=10, "Disabled"=15] ("Control Mode")
              n110 = call <vilib>:"CTRE_Phoenix_MotorControl_RefNumRegistryGet.vi"("refnum name"="elevador") -> ("error out"=w455:errorcluster, "PhoenixMotorControlDevRef"=w456:T3)  [unwired: 9 in]
              n111 = call <vilib>:"CTRE_Phoenix_MotorControl_Set.vi"("error in (no error)"=w455, "Output"=0.0, "Control Mode"=w454, "PhoenixMotorControlDevRef"=w456) -> ()  [unwired: 6 in, 2 out]
            }
            frame True {
              w460 = T9 0 items=["PercentOutput"=0, "Position"=1, "Velocity"=2, "Current"=3, "Follower"=5, "MotionProfile"=6, "MotionMagic"=7, "MotionProfileArc"=10, "Disabled"=15] ("Control Mode")
              n112 = Negate(x=w457) -> (-x=w458:dbl)
              n113 = call <vilib>:"CTRE_Phoenix_MotorControl_RefNumRegistryGet.vi"("refnum name"="elevador") -> ("error out"=w461:errorcluster, "PhoenixMotorControlDevRef"=w462:T3)  [unwired: 9 in]
              n114 = call <vilib>:"CTRE_Phoenix_MotorControl_Set.vi"("error in (no error)"=w461, "Output"=w458, "Control Mode"=w460, "PhoenixMotorControlDevRef"=w462) -> ()  [unwired: 6 in, 2 out]
            }
          }
        }
        frame True {
          n115 = local read "Disp_Valido"() -> (w465:dbl)
          n116 = Greater?(x=w465, y=10.0) -> (0:w466:bool)
          n117 = case shown="True" w466 {
            tunnel: 1.0 ("Output") -> [_ w472]
            frame False {
              w469 = T9 0 items=["PercentOutput"=0, "Position"=1, "Velocity"=2, "Current"=3, "Follower"=5, "MotionProfile"=6, "MotionMagic"=7, "MotionProfileArc"=10, "Disabled"=15] ("Control Mode")
              n118 = call <vilib>:"CTRE_Phoenix_MotorControl_RefNumRegistryGet.vi"("refnum name"="elevador") -> ("error out"=w470:errorcluster, "PhoenixMotorControlDevRef"=w471:T3)  [unwired: 9 in]
              n119 = call <vilib>:"CTRE_Phoenix_MotorControl_Set.vi"("error in (no error)"=w470, "Output"=0.0, "Control Mode"=w469, "PhoenixMotorControlDevRef"=w471) -> ()  [unwired: 6 in, 2 out]
            }
            frame True {
              w474 = T9 0 items=["PercentOutput"=0, "Position"=1, "Velocity"=2, "Current"=3, "Follower"=5, "MotionProfile"=6, "MotionMagic"=7, "MotionProfileArc"=10, "Disabled"=15] ("Control Mode")
              n120 = call <vilib>:"CTRE_Phoenix_MotorControl_RefNumRegistryGet.vi"("refnum name"="elevador") -> ("error out"=w475:errorcluster, "PhoenixMotorControlDevRef"=w476:T3)  [unwired: 9 in]
              n121 = call <vilib>:"CTRE_Phoenix_MotorControl_Set.vi"("error in (no error)"=w475, "Output"=w472, "Control Mode"=w474, "PhoenixMotorControlDevRef"=w476) -> ()  [unwired: 6 in, 2 out]
            }
          }
        }
      }
    }
  }
  n122 = case shown="True" w241 {
    tunnel: w244 -> [_ w483]
    frame False {
      w478 = T9 0 items=["PercentOutput"=0, "Position"=1, "Velocity"=2, "Current"=3, "Follower"=5, "MotionProfile"=6, "MotionMagic"=7, "MotionProfileArc"=10, "Disabled"=15] ("Control Mode")
      n123 = call <vilib>:"CTRE_Phoenix_MotorControl_RefNumRegistryGet.vi"("refnum name"="elevador") -> ("error out"=w480:errorcluster, "PhoenixMotorControlDevRef"=w481:T3)  [unwired: 9 in]
      n124 = call <vilib>:"CTRE_Phoenix_MotorControl_Set.vi"("error in (no error)"=w480, "Output"=0.0, "Control Mode"=w478, "PhoenixMotorControlDevRef"=w481) -> ()  [unwired: 6 in, 2 out]
    }
    frame True {
      n125 = Equal?(x=w483, y=i16 0) -> (x = y?=w484:bool)
      n126 = case shown="False" w484 {
        tunnel: w483 -> [w487 _]
        tunnel: 0.4 ("Output") -> [w486 _]
        frame False {
          n127 = Equal?(x=w487, y=180.0) -> (x = y?=w489:bool)
          n128 = case shown="True" w489 {
            tunnel: w486 -> [_ w495]
            frame False {
              w492 = T9 0 items=["PercentOutput"=0, "Position"=1, "Velocity"=2, "Current"=3, "Follower"=5, "MotionProfile"=6, "MotionMagic"=7, "MotionProfileArc"=10, "Disabled"=15] ("Control Mode")
              n129 = call <vilib>:"CTRE_Phoenix_MotorControl_RefNumRegistryGet.vi"("refnum name"="elevador") -> ("error out"=w493:errorcluster, "PhoenixMotorControlDevRef"=w494:T3)  [unwired: 9 in]
              n130 = call <vilib>:"CTRE_Phoenix_MotorControl_Set.vi"("error in (no error)"=w493, "Output"=0.0, "Control Mode"=w492, "PhoenixMotorControlDevRef"=w494) -> ()  [unwired: 6 in, 2 out]
            }
            frame True {
              w498 = T9 0 items=["PercentOutput"=0, "Position"=1, "Velocity"=2, "Current"=3, "Follower"=5, "MotionProfile"=6, "MotionMagic"=7, "MotionProfileArc"=10, "Disabled"=15] ("Control Mode")
              # "inverte o giro do motor para descer"
              n131 = Negate(x=w495) -> (-x=w496:dbl)
              n132 = call <vilib>:"CTRE_Phoenix_MotorControl_RefNumRegistryGet.vi"("refnum name"="elevador") -> ("error out"=w499:errorcluster, "PhoenixMotorControlDevRef"=w500:T3)  [unwired: 9 in]
              n133 = call <vilib>:"CTRE_Phoenix_MotorControl_Set.vi"("error in (no error)"=w499, "Output"=w496, "Control Mode"=w498, "PhoenixMotorControlDevRef"=w500) -> ()  [unwired: 6 in, 2 out]
            }
          }
        }
        frame True {
          n134 = global read "GlobalVariables.vi" "Disp_Valido"() -> (w501:dbl)
          n135 = Greater?(x=w501, y=10.0) -> (0:w504:bool)
          n136 = case shown="True" w504 {
            tunnel: 1.0 ("Output") -> [_ w510]
            frame False {
              w507 = T9 0 items=["PercentOutput"=0, "Position"=1, "Velocity"=2, "Current"=3, "Follower"=5, "MotionProfile"=6, "MotionMagic"=7, "MotionProfileArc"=10, "Disabled"=15] ("Control Mode")
              n137 = call <vilib>:"CTRE_Phoenix_MotorControl_RefNumRegistryGet.vi"("refnum name"="elevador") -> ("error out"=w508:errorcluster, "PhoenixMotorControlDevRef"=w509:T3)  [unwired: 9 in]
              n138 = call <vilib>:"CTRE_Phoenix_MotorControl_Set.vi"("error in (no error)"=w508, "Output"=0.0, "Control Mode"=w507, "PhoenixMotorControlDevRef"=w509) -> ()  [unwired: 6 in, 2 out]
            }
            frame True {
              w512 = T9 0 items=["PercentOutput"=0, "Position"=1, "Velocity"=2, "Current"=3, "Follower"=5, "MotionProfile"=6, "MotionMagic"=7, "MotionProfileArc"=10, "Disabled"=15] ("Control Mode")
              n139 = call <vilib>:"CTRE_Phoenix_MotorControl_RefNumRegistryGet.vi"("refnum name"="elevador") -> ("error out"=w513:errorcluster, "PhoenixMotorControlDevRef"=w514:T3)  [unwired: 9 in]
              n140 = call <vilib>:"CTRE_Phoenix_MotorControl_Set.vi"("error in (no error)"=w513, "Output"=w510, "Control Mode"=w512, "PhoenixMotorControlDevRef"=w514) -> ()  [unwired: 6 in, 2 out]
            }
          }
        }
      }
    }
  }
  n141 = global read "GlobalVariables.vi" "Pos_Braco"() -> (w11:dbl)
  n142 = call <vilib>:"WPI_EncoderRefNum Registry Get.vi"("refnum name"="EncBraco") -> ("error out"=w17:errorcluster, "EncoderDevRef"=w14:T15)  [unwired: 9 in]
  n143 = global read "GlobalVariables.vi" "Aim_Lock"() -> (w237:bool)
  n144 = feedback #1(FALSE) -> (w28:bool)
  n145 = case shown="False" w26 {
    selector: w26 -> [_ w531]
    tunnel: w28 -> [w518 w533]
    tunnel: [w519 w532] -> w27
    frame False {
      # "loop numerico de dados"
      n146 = feedback #2(0.0) -> (w515:dbl)
      n147 = case shown="True" w518 {
        selector: w518 -> [w521 w522]
        tunnel: [w521 w527] -> w519
        tunnel: [0.0 w523] -> w516
        tunnel: w515 -> [_ w524]
        frame False {
        }
        frame True {
          # "delay de 800ms"
          n148 = Increment(x=w524) -> (x+1=w523:dbl)
          n149 = Greater?(x=w523, y=20.0) -> (0:w526:bool)
          n150 = case shown="True" w526 {
            tunnel: [w528 w529] -> w527
            tunnel: w522 -> [w528 _]
            frame False {
            }
            frame True {
              w529 = FALSE
              # "Variável local para interromper a o PID"
              n151 = global read "GlobalVariables.vi" "Dist_Braco"() -> (w530:dbl)
              n152 = local write "Stop_pid"(w529) -> ()
              n153 = global write "GlobalVariables.vi" "Pos_Braco"(w530) -> ()
            }
          }
        }
      }
      n154 = feedback-in #2(w516) -> ()
    }
    frame True {
      n155 = local write "Stop_pid"(w531) -> ()
      n156 = case shown="True" w533 {
        selector: w533 -> [_ w535]
        tunnel: [TRUE w535] -> w532
        frame False {
        }
        frame True {
        }
      }
      "Stop_pid" <- w531
    }
  }
  n157 = feedback-in #1(w27) -> ()
  n158 = Not(x="Stop_PID") -> (.not. x?=w6:bool)
  n159 = local read "Lime_Min"() -> (w287:dbl)
  n160 = call "Vi_por_infeite_deletar_depois.vi"() -> ("Boolean"=w220:bool)  [unwired: 9 in, 2 out]
  n161 = call <vilib>:"WPI_EncoderConfigureTimer.vi"("error in (no error)"=w17, "Number Samples to Average"=u8 3, "Minimum Rate"=20.0, "EncoderDevRef"=w14) -> ("error out"=w16:errorcluster, "EncoderDevRef"=w15:T15)  [unwired: 6 in]
  n162 = Wait (ms)(milliseconds to wait=40) -> ()  [unwired: 1 out]
  n163 = call <vilib>:"WPI_EncoderGet.vi"("error in (no error)"=w16, "EncoderDevRef"=w15) -> ("Distance"=w10:dbl)  [unwired: 4 in, 5 out]
  "Distance" <- w10
  n164 = call <vilib>:"WPI_JoystickRefNum Registry Get.vi"("refnum name"="Joystick 0") -> ("JoystickDevRef"=w266:T11)  [unwired: 1 in, 9 out]
  n165 = case shown="True" w237 {
    frame False {
      w537 = T9 0 items=["PercentOutput"=0, "Position"=1, "Velocity"=2, "Current"=3, "Follower"=5, "MotionProfile"=6, "MotionMagic"=7, "MotionProfileArc"=10, "Disabled"=15] ("Control Mode")
      n166 = call <vilib>:"CTRE_Phoenix_MotorControl_RefNumRegistryGet.vi"("refnum name"="disparador") -> ("error out"=w538:errorcluster, "PhoenixMotorControlDevRef"=w539:T3)  [unwired: 9 in]
      n167 = call <vilib>:"CTRE_Phoenix_MotorControl_Set.vi"("error in (no error)"=w538, "Output"=0.0, "Control Mode"=w537, "PhoenixMotorControlDevRef"=w539) -> ()  [unwired: 6 in, 2 out]
    }
    frame True {
      w546 = T9 0 items=["PercentOutput"=0, "Position"=1, "Velocity"=2, "Current"=3, "Follower"=5, "MotionProfile"=6, "MotionMagic"=7, "MotionProfileArc"=10, "Disabled"=15] ("Control Mode")
      # "Velocidade controlada através do eixo 2 e 3 (gatilhos L1 e R1)"
      n168 = call <vilib>:"WPI_JoystickRefNum Registry Get.vi"("refnum name"="Joystick 0") -> ("error out"=w553:errorcluster, "JoystickDevRef"=w552:T11)  [unwired: 1 in, 8 out]
      n169 = call <vilib>:"WPI_JoystickGetValues.vi"("error in (no error)"=w553, "JoystickDevRef"=w552) -> ("Axes"=w550:dbl[])  [unwired: 5 in, 4 out]
      n170 = Array To Cluster(array=w550) -> (cluster=w549:T19)
      n171 = Unbundle By Name(w549) -> ("Axes[2]"=w542:dbl, "Axes[3]"=w543:dbl)
      n172 = Negate(x=w543) -> (-x=w544:dbl)
      n173 = Add(x=w542, y=w544) -> (x+y=w541:dbl)
      "pwm_shot" <- w541
      n174 = call <vilib>:"CTRE_Phoenix_MotorControl_RefNumRegistryGet.vi"("refnum name"="disparador") -> ("error out"=w545:errorcluster, "PhoenixMotorControlDevRef"=w547:T3)  [unwired: 9 in]
      n175 = call <vilib>:"CTRE_Phoenix_MotorControl_Set.vi"("error in (no error)"=w545, "Output"=w541, "Control Mode"=w546, "PhoenixMotorControlDevRef"=w547) -> ()  [unwired: 6 in, 2 out]
    }
  }
  n176 = case shown="True" w220 {
    frame False {
      w557 = T9 0 items=["PercentOutput"=0, "Position"=1, "Velocity"=2, "Current"=3, "Follower"=5, "MotionProfile"=6, "MotionMagic"=7, "MotionProfileArc"=10, "Disabled"=15] ("Control Mode")
      n177 = call <vilib>:"CTRE_Phoenix_MotorControl_RefNumRegistryGet.vi"("refnum name"="elevador_total") -> ("error out"=w556:errorcluster, "PhoenixMotorControlDevRef"=w555:T3)  [unwired: 9 in]
      n178 = call <vilib>:"CTRE_Phoenix_MotorControl_Set.vi"("error in (no error)"=w556, "Output"=0.0, "Control Mode"=w557, "PhoenixMotorControlDevRef"=w555) -> ()  [unwired: 6 in, 2 out]
    }
    frame True {
      w561 = T9 0 items=["PercentOutput"=0, "Position"=1, "Velocity"=2, "Current"=3, "Follower"=5, "MotionProfile"=6, "MotionMagic"=7, "MotionProfileArc"=10, "Disabled"=15] ("Control Mode")
      # "Eixo que move o elevador do robô para cima ou para baixo."
      n179 = call <vilib>:"WPI_JoystickRefNum Registry Get.vi"("refnum name"="Joystick 0") -> ("JoystickDevRef"=w566:T11)  [unwired: 1 in, 9 out]
      n180 = call <vilib>:"WPI_JoystickGetValues.vi"("JoystickDevRef"=w566) -> ("Axes"=w564:dbl[])  [unwired: 6 in, 4 out]
      n181 = Array To Cluster(array=w564) -> (cluster=w565:T20)
      n182 = Unbundle By Name(w565) -> ("Axes[5]"=w559:dbl)
      n183 = call <vilib>:"CTRE_Phoenix_MotorControl_RefNumRegistryGet.vi"("refnum name"="elevador_total") -> ("error out"=w563:errorcluster, "PhoenixMotorControlDevRef"=w562:T3)  [unwired: 9 in]
      n184 = call <vilib>:"CTRE_Phoenix_MotorControl_Set.vi"("error in (no error)"=w563, "Output"=w559, "Control Mode"=w561, "PhoenixMotorControlDevRef"=w562) -> ()  [unwired: 6 in, 2 out]
    }
  }
  n185 = feedback #3(0.6 ("y")) -> (w205:dbl)
  n186 = feedback #4(0.6 ("y")) -> (w142:dbl)
  n187 = case shown="False" w245 {
    tunnel: w246 -> [w568 _]
    frame False {
      n188 = case shown="True" w568 {
        tunnel: 0.5 ("Output") -> [_ w576]
        frame False {
          w571 = T9 0 items=["PercentOutput"=0, "Position"=1, "Velocity"=2, "Current"=3, "Follower"=5, "MotionProfile"=6, "MotionMagic"=7, "MotionProfileArc"=10, "Disabled"=15] ("Control Mode")
          n189 = call <vilib>:"CTRE_Phoenix_MotorControl_RefNumRegistryGet.vi"("refnum name"="abraco") -> ("error out"=w573:errorcluster, "PhoenixMotorControlDevRef"=w574:T3)  [unwired: 9 in]
          n190 = call <vilib>:"CTRE_Phoenix_MotorControl_Set.vi"("error in (no error)"=w573, "Output"=0.0, "Control Mode"=w571, "PhoenixMotorControlDevRef"=w574) -> ()  [unwired: 6 in, 2 out]
        }
        frame True {
          w577 = T9 0 items=["PercentOutput"=0, "Position"=1, "Velocity"=2, "Current"=3, "Follower"=5, "MotionProfile"=6, "MotionMagic"=7, "MotionProfileArc"=10, "Disabled"=15] ("Control Mode")
          n191 = Negate(x=w576) -> (-x=w575:dbl)
          n192 = call <vilib>:"CTRE_Phoenix_MotorControl_RefNumRegistryGet.vi"("refnum name"="abraco") -> ("error out"=w579:errorcluster, "PhoenixMotorControlDevRef"=w578:T3)  [unwired: 9 in]
          n193 = call <vilib>:"CTRE_Phoenix_MotorControl_Set.vi"("error in (no error)"=w579, "Output"=w575, "Control Mode"=w577, "PhoenixMotorControlDevRef"=w578) -> ()  [unwired: 6 in, 2 out]
        }
      }
    }
    frame True {
      w581 = T9 0 items=["PercentOutput"=0, "Position"=1, "Velocity"=2, "Current"=3, "Follower"=5, "MotionProfile"=6, "MotionMagic"=7, "MotionProfileArc"=10, "Disabled"=15] ("Control Mode")
      n194 = call <vilib>:"CTRE_Phoenix_MotorControl_RefNumRegistryGet.vi"("refnum name"="abraco") -> ("error out"=w583:errorcluster, "PhoenixMotorControlDevRef"=w584:T3)  [unwired: 9 in]
      n195 = call <vilib>:"CTRE_Phoenix_MotorControl_Set.vi"("error in (no error)"=w583, "Output"=0.5, "Control Mode"=w581, "PhoenixMotorControlDevRef"=w584) -> ()  [unwired: 6 in, 2 out]
    }
  }
  n196 = case shown="True" w248 {
    selector: w248 -> [_ w600]
    tunnel: w247 -> [w586 _]
    frame False {
      # "Expulsar"
      n197 = case shown="False" w586 {
        tunnel: 0.9 -> [_ w594]
        frame False {
          w589 = T9 0 items=["PercentOutput"=0, "Position"=1, "Velocity"=2, "Current"=3, "Follower"=5, "MotionProfile"=6, "MotionMagic"=7, "MotionProfileArc"=10, "Disabled"=15] ("Control Mode")
          n198 = call <vilib>:"CTRE_Phoenix_MotorControl_RefNumRegistryGet.vi"("refnum name"="braco") -> ("error out"=w592:errorcluster, "PhoenixMotorControlDevRef"=w591:T3)  [unwired: 9 in]
          n199 = call <vilib>:"CTRE_Phoenix_MotorControl_Set.vi"("error in (no error)"=w592, "Output"=0.0, "Control Mode"=w589, "PhoenixMotorControlDevRef"=w591) -> ()  [unwired: 6 in, 2 out]
        }
        frame True {
          w596 = T9 0 items=["PercentOutput"=0, "Position"=1, "Velocity"=2, "Current"=3, "Follower"=5, "MotionProfile"=6, "MotionMagic"=7, "MotionProfileArc"=10, "Disabled"=15] ("Control Mode")
          n200 = Negate(x=w594) -> (-x=w593:dbl)
          n201 = call <vilib>:"CTRE_Phoenix_MotorControl_RefNumRegistryGet.vi"("refnum name"="braco") -> ("error out"=w597:errorcluster, "PhoenixMotorControlDevRef"=w598:T3)  [unwired: 9 in]
          n202 = call <vilib>:"CTRE_Phoenix_MotorControl_Set.vi"("error in (no error)"=w597, "Output"=w593, "Control Mode"=w596, "PhoenixMotorControlDevRef"=w598) -> ()  [unwired: 6 in, 2 out]
        }
      }
    }
    frame True {
      n203 = case shown="True" w600 {
        tunnel: 1.0 ("Output") -> [_ w608]
        frame False {
          w602 = T9 0 items=["PercentOutput"=0, "Position"=1, "Velocity"=2, "Current"=3, "Follower"=5, "MotionProfile"=6, "MotionMagic"=7, "MotionProfileArc"=10, "Disabled"=15] ("Control Mode")
          n204 = call <vilib>:"CTRE_Phoenix_MotorControl_RefNumRegistryGet.vi"("refnum name"="braco") -> ("error out"=w605:errorcluster, "PhoenixMotorControlDevRef"=w604:T3)  [unwired: 9 in]
          n205 = call <vilib>:"CTRE_Phoenix_MotorControl_Set.vi"("error in (no error)"=w605, "Output"=0.0, "Control Mode"=w602, "PhoenixMotorControlDevRef"=w604) -> ()  [unwired: 6 in, 2 out]
        }
        frame True {
          w607 = T9 0 items=["PercentOutput"=0, "Position"=1, "Velocity"=2, "Current"=3, "Follower"=5, "MotionProfile"=6, "MotionMagic"=7, "MotionProfileArc"=10, "Disabled"=15] ("Control Mode")
          n206 = call <vilib>:"CTRE_Phoenix_MotorControl_RefNumRegistryGet.vi"("refnum name"="braco") -> ("error out"=w609:errorcluster, "PhoenixMotorControlDevRef"=w610:T3)  [unwired: 9 in]
          n207 = call <vilib>:"CTRE_Phoenix_MotorControl_Set.vi"("error in (no error)"=w609, "Output"=w608, "Control Mode"=w607, "PhoenixMotorControlDevRef"=w610) -> ()  [unwired: 6 in, 2 out]
        }
      }
    }
  }
  n208 = Subtract(x="Mot_Max", y="Mot_Min") -> (x-y=w294:dbl)
  n209 = Subtract(x=w281, y=w287) -> (x-y=w293:dbl)
  n210 = xnode "PID"("setpoint"=w11, "process variable"=w10, "proportional gain (Kc)"=0.01, "integral time (Ti, min)"=0.09, "derivative time (Td, min)"=0.0001, "auto? (T)"=w6, "output high"=0.25, "output low"=-0.25) -> ("output"=w25:dbl)  [unwired: 1 in, 1 out]
  "pidOut" <- w25
  n211 = feedback #5(FALSE) -> (w214:bool)
  n212 = local read "Lime_Max"() -> (w286:dbl)
  n213 = feedback #6(FALSE) -> (w133:bool)
  n214 = call <vilib>:"WPI_JoystickGetValues.vi"("JoystickDevRef"=w266) -> ("Axes"=w268:dbl[])  [unwired: 6 in, 4 out]
  n215 = global write "GlobalVariables.vi" "Dist_Braco"(w10) -> ()
  n216 = call <vilib>:"WPI_JoystickRefNum Registry Get.vi"("refnum name"="Joystick 0") -> ("JoystickDevRef"=w317:T11)  [unwired: 1 in, 9 out]
  n217 = local read "pwm_shot"() -> (w235:dbl)
  n218 = case shown="False" {
    selector: _ -> [_ w624]
    frame False {
      # "Expulsar"
      n219 = case shown="False" {
        selector: _ -> [_ _]
        tunnel: 0.9 -> [_ w618]
        frame False {
          w613 = T9 0 items=["PercentOutput"=0, "Position"=1, "Velocity"=2, "Current"=3, "Follower"=5, "MotionProfile"=6, "MotionMagic"=7, "MotionProfileArc"=10, "Disabled"=15] ("Control Mode")
          n220 = call <vilib>:"CTRE_Phoenix_MotorControl_RefNumRegistryGet.vi"("refnum name"="braco") -> ("error out"=w616:errorcluster, "PhoenixMotorControlDevRef"=w615:T3)  [unwired: 9 in]
          n221 = call <vilib>:"CTRE_Phoenix_MotorControl_Set.vi"("error in (no error)"=w616, "Output"=0.0, "Control Mode"=w613, "PhoenixMotorControlDevRef"=w615) -> ()  [unwired: 6 in, 2 out]
        }
        frame True {
          w620 = T9 0 items=["PercentOutput"=0, "Position"=1, "Velocity"=2, "Current"=3, "Follower"=5, "MotionProfile"=6, "MotionMagic"=7, "MotionProfileArc"=10, "Disabled"=15] ("Control Mode")
          n222 = Negate(x=w618) -> (-x=w617:dbl)
          n223 = call <vilib>:"CTRE_Phoenix_MotorControl_RefNumRegistryGet.vi"("refnum name"="braco") -> ("error out"=w621:errorcluster, "PhoenixMotorControlDevRef"=w622:T3)  [unwired: 9 in]
          n224 = call <vilib>:"CTRE_Phoenix_MotorControl_Set.vi"("error in (no error)"=w621, "Output"=w617, "Control Mode"=w620, "PhoenixMotorControlDevRef"=w622) -> ()  [unwired: 6 in, 2 out]
        }
      }
    }
    frame True {
      n225 = case shown="True" w624 {
        tunnel: 1.0 ("Output") -> [_ w632]
        frame False {
          w626 = T9 0 items=["PercentOutput"=0, "Position"=1, "Velocity"=2, "Current"=3, "Follower"=5, "MotionProfile"=6, "MotionMagic"=7, "MotionProfileArc"=10, "Disabled"=15] ("Control Mode")
          n226 = call <vilib>:"CTRE_Phoenix_MotorControl_RefNumRegistryGet.vi"("refnum name"="braco") -> ("error out"=w629:errorcluster, "PhoenixMotorControlDevRef"=w628:T3)  [unwired: 9 in]
          n227 = call <vilib>:"CTRE_Phoenix_MotorControl_Set.vi"("error in (no error)"=w629, "Output"=0.0, "Control Mode"=w626, "PhoenixMotorControlDevRef"=w628) -> ()  [unwired: 6 in, 2 out]
        }
        frame True {
          w631 = T9 0 items=["PercentOutput"=0, "Position"=1, "Velocity"=2, "Current"=3, "Follower"=5, "MotionProfile"=6, "MotionMagic"=7, "MotionProfileArc"=10, "Disabled"=15] ("Control Mode")
          n228 = call <vilib>:"CTRE_Phoenix_MotorControl_RefNumRegistryGet.vi"("refnum name"="braco") -> ("error out"=w633:errorcluster, "PhoenixMotorControlDevRef"=w634:T3)  [unwired: 9 in]
          n229 = call <vilib>:"CTRE_Phoenix_MotorControl_Set.vi"("error in (no error)"=w633, "Output"=w632, "Control Mode"=w631, "PhoenixMotorControlDevRef"=w634) -> ()  [unwired: 6 in, 2 out]
        }
      }
    }
  }
  n230 = case shown="False" {
    selector: _ -> [_ w648]
    frame False {
      # "Expulsar"
      n231 = case shown="False" {
        selector: _ -> [_ _]
        tunnel: 0.9 -> [_ w642]
        frame False {
          w637 = T9 0 items=["PercentOutput"=0, "Position"=1, "Velocity"=2, "Current"=3, "Follower"=5, "MotionProfile"=6, "MotionMagic"=7, "MotionProfileArc"=10, "Disabled"=15] ("Control Mode")
          n232 = call <vilib>:"CTRE_Phoenix_MotorControl_RefNumRegistryGet.vi"("refnum name"="braco") -> ("error out"=w640:errorcluster, "PhoenixMotorControlDevRef"=w639:T3)  [unwired: 9 in]
          n233 = call <vilib>:"CTRE_Phoenix_MotorControl_Set.vi"("error in (no error)"=w640, "Output"=0.0, "Control Mode"=w637, "PhoenixMotorControlDevRef"=w639) -> ()  [unwired: 6 in, 2 out]
        }
        frame True {
          w644 = T9 0 items=["PercentOutput"=0, "Position"=1, "Velocity"=2, "Current"=3, "Follower"=5, "MotionProfile"=6, "MotionMagic"=7, "MotionProfileArc"=10, "Disabled"=15] ("Control Mode")
          n234 = Negate(x=w642) -> (-x=w641:dbl)
          n235 = call <vilib>:"CTRE_Phoenix_MotorControl_RefNumRegistryGet.vi"("refnum name"="braco") -> ("error out"=w645:errorcluster, "PhoenixMotorControlDevRef"=w646:T3)  [unwired: 9 in]
          n236 = call <vilib>:"CTRE_Phoenix_MotorControl_Set.vi"("error in (no error)"=w645, "Output"=w641, "Control Mode"=w644, "PhoenixMotorControlDevRef"=w646) -> ()  [unwired: 6 in, 2 out]
        }
      }
    }
    frame True {
      n237 = case shown="True" w648 {
        tunnel: 1.0 ("Output") -> [_ w656]
        frame False {
          w650 = T9 0 items=["PercentOutput"=0, "Position"=1, "Velocity"=2, "Current"=3, "Follower"=5, "MotionProfile"=6, "MotionMagic"=7, "MotionProfileArc"=10, "Disabled"=15] ("Control Mode")
          n238 = call <vilib>:"CTRE_Phoenix_MotorControl_RefNumRegistryGet.vi"("refnum name"="braco") -> ("error out"=w653:errorcluster, "PhoenixMotorControlDevRef"=w652:T3)  [unwired: 9 in]
          n239 = call <vilib>:"CTRE_Phoenix_MotorControl_Set.vi"("error in (no error)"=w653, "Output"=0.0, "Control Mode"=w650, "PhoenixMotorControlDevRef"=w652) -> ()  [unwired: 6 in, 2 out]
        }
        frame True {
          w655 = T9 0 items=["PercentOutput"=0, "Position"=1, "Velocity"=2, "Current"=3, "Follower"=5, "MotionProfile"=6, "MotionMagic"=7, "MotionProfileArc"=10, "Disabled"=15] ("Control Mode")
          n240 = call <vilib>:"CTRE_Phoenix_MotorControl_RefNumRegistryGet.vi"("refnum name"="braco") -> ("error out"=w657:errorcluster, "PhoenixMotorControlDevRef"=w658:T3)  [unwired: 9 in]
          n241 = call <vilib>:"CTRE_Phoenix_MotorControl_Set.vi"("error in (no error)"=w657, "Output"=w656, "Control Mode"=w655, "PhoenixMotorControlDevRef"=w658) -> ()  [unwired: 6 in, 2 out]
        }
      }
    }
  }
  n242 = Array To Cluster(array=w268) -> (cluster=w269:T1)
  n243 = Multiply(x=w294, y=w293) -> (x*y=w292:dbl)
  n244 = feedback #7(FALSE) -> (w212:bool)
  n245 = case shown="True" w217 {
    tunnel: w218 -> [w665 _]
    tunnel: [w663 w685] -> w203
    tunnel: w205 -> [w664 w686]
    tunnel: w214 -> [w662 w687]
    tunnel: [w661 w684] -> w213
    tunnel: w212 -> [w660 w683]
    tunnel: [w659 w683] -> w211
    frame False {
      n246 = case shown="True" w665 {
        tunnel: w664 -> [w670 w676]
        tunnel: [w670 w675] -> w663
        tunnel: w660 -> [w669 w674]
        tunnel: [w668 w673] -> w659
        frame False {
          n247 = case shown="False" w669 {
            selector: w669 -> [w671 _]
            tunnel: [w671 FALSE] -> w668
            frame False {
            }
            frame True {
            }
          }
        }
        frame True {
          n248 = case shown="False" w674 {
            selector: w674 -> [_ w681]
            tunnel: w676 -> [w679 w682]
            tunnel: [w678 w682] -> w675
            tunnel: [TRUE w681] -> w673
            frame False {
              # "redutor de \nvelocidadde"
              n249 = Subtract(x=w679, y=0.2) -> (x-y=w678:dbl)
            }
            frame True {
            }
          }
        }
      }
      n250 = case shown="False" w662 {
        selector: w662 -> [w666 _]
        tunnel: [w666 FALSE] -> w661
        frame False {
        }
        frame True {
        }
      }
    }
    frame True {
      n251 = case shown="False" w687 {
        selector: w687 -> [_ w692]
        tunnel: w686 -> [w690 w693]
        tunnel: [w689 w693] -> w685
        tunnel: [TRUE w692] -> w684
        frame False {
          # "incrementar \nvelocidade."
          n252 = Add(x=w690, y=0.2) -> (x+y=w689:dbl)
        }
        frame True {
        }
      }
    }
  }
  "Multiplicação 3" <- w203
  n253 = feedback-in #5(w213) -> ()
  n254 = feedback-in #7(w211) -> ()
  n255 = feedback #8(FALSE) -> (w135:bool)
  n256 = case shown="False" w130 {
    tunnel: w129 -> [w700 _]
    tunnel: [w698 w720] -> w144
    tunnel: w142 -> [w699 w721]
    tunnel: w133 -> [w697 w722]
    tunnel: [w696 w719] -> w134
    tunnel: w135 -> [w695 w718]
    tunnel: [w694 w718] -> w136
    frame False {
      n257 = case shown="True" w700 {
        tunnel: w699 -> [w705 w711]
        tunnel: [w705 w710] -> w698
        tunnel: w695 -> [w704 w709]
        tunnel: [w703 w708] -> w694
        frame False {
          n258 = case shown="False" w704 {
            selector: w704 -> [w706 _]
            tunnel: [w706 FALSE] -> w703
            frame False {
            }
            frame True {
            }
          }
        }
        frame True {
          n259 = case shown="False" w709 {
            selector: w709 -> [_ w716]
            tunnel: w711 -> [w714 w717]
            tunnel: [w713 w717] -> w710
            tunnel: [TRUE w716] -> w708
            frame False {
              # "redutor de \nvelocidadde"
              n260 = Subtract(x=w714, y=0.2) -> (x-y=w713:dbl)
            }
            frame True {
            }
          }
        }
      }
      n261 = case shown="False" w697 {
        selector: w697 -> [w701 _]
        tunnel: [w701 FALSE] -> w696
        frame False {
        }
        frame True {
        }
      }
    }
    frame True {
      n262 = case shown="False" w722 {
        selector: w722 -> [_ w727]
        tunnel: w721 -> [w725 w728]
        tunnel: [w724 w728] -> w720
        tunnel: [TRUE w727] -> w719
        frame False {
          # "incrementar \nvelocidade."
          n263 = Add(x=w725, y=0.2) -> (x+y=w724:dbl)
        }
        frame True {
        }
      }
    }
  }
  "Multiplicação 6" <- w144
  n264 = feedback-in #6(w134) -> ()
  n265 = feedback-in #8(w136) -> ()
  n266 = call <vilib>:"WPI_JoystickGetValues.vi"("JoystickDevRef"=w317) -> ("Axes"=w319:dbl[])  [unwired: 6 in, 4 out]
  n267 = call <vilib>:"WPI_JoystickRefNum Registry Get.vi"("refnum name"="Joystick 0") -> ("JoystickDevRef"=w332:T11)  [unwired: 1 in, 9 out]
  n268 = Subtract(x=w286, y=w287) -> (x-y=w291:dbl)
  n269 = Array To Cluster(array=w319) -> (cluster=w320:T1)
  n270 = Absolute Value(x=w235) -> (abs(x)=w234:dbl)
  n271 = call <vilib>:"WPI_JoystickGetValues.vi"("JoystickDevRef"=w332) -> ("Axes"=w330:dbl[])  [unwired: 6 in, 4 out]
  n272 = feedback #9(FALSE) -> (w224:bool)
  n273 = Unbundle By Name(w269) -> ("Axes[1]"=w264:dbl, "Axes[2]"=w263:dbl, "Axes[3]"=w262:dbl, "Axes[4]"=w261:dbl)
  n274 = global read "GlobalVariables.vi" "Aim_Lock"() -> (w232:bool)
  n275 = feedback #10(FALSE) -> (w222:bool)
  n276 = case shown="False" w202 {
    tunnel: [w732 w740] -> w226
    tunnel: w224 -> [w729 w741]
    tunnel: w222 -> [w731 w739]
    tunnel: [w730 w738] -> w221
    frame False {
      n277 = case shown="False" w731 {
        selector: w731 -> [w734 w737]
        tunnel: [w733 w735] -> w732
        tunnel: [w734 w736] -> w730
        tunnel: w729 -> [w733 w735]
        frame False {
        }
        frame True {
          n278 = Not(x=w737) -> (.not. x?=w736:bool)
        }
      }
    }
    frame True {
      n279 = case shown="False" w739 {
        selector: w739 -> [_ w745]
        tunnel: w741 -> [w743 w746]
        tunnel: [w744 w746] -> w740
        tunnel: [TRUE w745] -> w738
        frame False {
          n280 = Not(x=w743) -> (.not. x?=w744:bool)
        }
        frame True {
        }
      }
    }
  }
  "OUT_PUT" <- w226
  n281 = feedback-in #9(w226) -> ()
  n282 = feedback-in #10(w221) -> ()
  n283 = call <vilib>:"WPI_RobotDriveRefNum Registry Get.vi"("refnum name"="Left and Right Motors") -> ("error out"=w272:errorcluster, "RobotDriveDevRef"=w271:T2)  [unwired: 9 in]
  n284 = call <vilib>:"WPI_RobotDriveRefNum Registry Get.vi"("refnum name"="Left and Right Motors") -> ("error out"=w326:errorcluster, "RobotDriveDevRef"=w327:T2)  [unwired: 9 in]
  n285 = Array To Cluster(array=w330) -> (cluster=w329:T1)
  n286 = Greater?(x=w234, y=0.1) -> (0:w233:bool)
  n287 = And(x=w233, y=w232) -> (x .and. y?=w231:bool)
  n288 = Unbundle By Name(w320) -> ("Axes[0]"=w316:dbl, "Axes[1]"=w315:dbl, "Axes[2]"=w313:dbl, "Axes[3]"=w312:dbl)
  n289 = call <vilib>:"WPI_RobotDriveRefNum Registry Get.vi"("refnum name"="Left and Right Motors") -> ("error out"=w323:errorcluster, "RobotDriveDevRef"=w322:T2)  [unwired: 9 in]
  n290 = Add(x=w262, y=w261) -> (x+y=w260:dbl)
  n291 = Add(x=w264, y=w263) -> (x+y=w265:dbl)
  n292 = Unbundle By Name(w329) -> ("Axes[1]"=w325:dbl, "Axes[2]"=w324:dbl)
  n293 = call <vilib>:"CTRE_Phoenix_MotorControl_RefNumRegistryGet.vi"("refnum name"="abraco") -> ("error out"=w18:errorcluster, "PhoenixMotorControlDevRef"=w19:T3)  [unwired: 9 in]
  n294 = Divide(x=w292, y=w291) -> (x/y=w290:dbl)
  n295 = call "Vi_por_infeite_deletar_depois.vi"("Numeric"=w203) -> ("Numeric 3"=w204:dbl)  [unwired: 8 in, 2 out]
  "OUT 3" <- w204
  n296 = feedback-in #3(w204) -> ()
  n297 = call "Vi_por_infeite_deletar_depois.vi"("Numeric"=w144) -> ("Numeric 3"=w143:dbl)  [unwired: 8 in, 2 out]
  "OUT 6" <- w143
  n298 = feedback-in #4(w143) -> ()
  n299 = feedback #11(0.0) -> (w228:dbl)
  n300 = case shown="True" w231 {
    tunnel: [0.0 w749] -> w230
    tunnel: w228 -> [_ w748]
    frame False {
    }
    frame True {
      n301 = Increment(x=w748) -> (x+1=w749:dbl)
    }
  }
  "Disp_Valido" <- w230
  n302 = feedback-in #11(w230) -> ()
  n303 = call <vilib>:"CTRE_Phoenix_MotorControl_Set.vi"("error in (no error)"=w18, "Output"=w25, "Control Mode"=w20, "PhoenixMotorControlDevRef"=w19) -> ()  [unwired: 6 in, 2 out]
  n304 = Negate(x=w316) -> (-x=w314:dbl)
  n305 = call <vilib>:"WPI_RobotDriveRefNum Registry Get.vi"("refnum name"="Left and Right Motors") -> ("error out"=w298:errorcluster, "RobotDriveDevRef"=w300:T2)  [unwired: 9 in]
  n306 = local read "Negar"() -> (w280:bool)
  n307 = Add(x=w290, y="Mot_Min") -> (x+y=w279:dbl)
  n308 = Add(x=w313, y=w312) -> (x+y=w310:dbl)
  n309 = Add(x=w314, y=w315) -> (x+y=w311:dbl)
  n310 = call-poly <vilib>:"WPI_RobotDriveArcadeDrive.vi"("error in (no error)"=w298, "Y axis value"=w303, "X axis value"=w302, "RobotDriveDevRef"=w300) -> ("Motor Values"=→"Motor Values":dbl[], "RobotDriveDevRef"=→"RobotDriveDevRef":T2)  [unwired: 5 in, 1 out]
  n311 = case shown="True" w280 {
    tunnel: w279 -> [w750 w752]
    tunnel: [w750 w751] -> w278
    frame False {
    }
    frame True {
      n312 = Negate(x=w752) -> (-x=w751:dbl)
    }
  }
  "x+y" <- w278
  n313 = call-poly <vilib>:"WPI_RobotDriveArcadeDrive.vi"("error in (no error)"=w326, "Y axis value"=w324, "X axis value"=w325, "RobotDriveDevRef"=w327) -> ()  [unwired: 5 in, 3 out]
  n314 = call-poly <vilib>:"WPI_RobotDriveArcadeDrive.vi"("error in (no error)"=w323, "Y axis value"=w310, "X axis value"=w311, "RobotDriveDevRef"=w322) -> ()  [unwired: 5 in, 3 out]
  n315 = call-poly <vilib>:"WPI_RobotDriveArcadeDrive.vi"("error in (no error)"=w272, "Y axis value"=w260, "X axis value"=w265, "RobotDriveDevRef"=w271) -> ()  [unwired: 5 in, 3 out]
  n316 = while {
    stop <- FALSE stop-if-true
    # "code location:\nperiodic tasks.Vi"
    # "The global variable that will allow the code to work in other areas of the program."
    # "The Lime Light programming system \ncomes ready to use, just take it from the \nInternet and copy it into the code."
    # "vertical angle"
    # "Horizontal angle"
    # "limelight target"
    # "10 ms tasks go here"
    n317 = call-poly <vilib>:"NT Read Value.vi"("Name"="/limelight/tx") -> ("Numeric"=w755:dbl)  [unwired: 9 in, 1 out]
    n318 = call-poly <vilib>:"NT Read Value.vi"("Name"="/limelight/ty") -> ("Numeric"=w754:dbl)  [unwired: 9 in, 1 out]
    n319 = call-poly <vilib>:"NT Read Value.vi"("Name"="/limelight/ta") -> ("Numeric"=w762:dbl)  [unwired: 9 in, 1 out]
    n320 = call-poly <vilib>:"NT Read Value.vi"("Name"="/limelight/ts") -> ("Numeric"=w763:dbl)  [unwired: 9 in, 1 out]
    n321 = call-poly <vilib>:"NT Read Value.vi"("Name"="/limelight/tv") -> ("Numeric"=w756:dbl)  [unwired: 9 in, 1 out]
    n322 = Bundle By Name(cluster=T8 {"offsetAngle H"=0.0, "offsetAngle V"=0.0, "area"=0.0, "skew"=0.0, "ValidT"=0.0} ("input cluster"), "offsetAngle H"=w755, "offsetAngle V"=w754, "area"=w762, "skew"=w763, "ValidT"=w756) -> (→"output cluster 2":T8)
    n323 = Equal?(x=w756, y=1.0) -> (x = y?=w753:bool)
    n324 = global write "GlobalVariables.vi" "Tx"(w755) -> ()
    n325 = global write "GlobalVariables.vi" "Ty"(w754) -> ()
    n326 = global write "GlobalVariables.vi" "ValidTarget"(w753) -> ()
    n327 = Wait (ms)(milliseconds to wait=u32 10) -> ()  [unwired: 1 out]
  }
  n328 = call <vilib>:"WPI_JoystickRefNum Registry Get.vi"("refnum name"="Joystick 0") -> ("JoystickDevRef"=w55:T11)  [unwired: 1 in, 9 out]
  n329 = case shown="True" {
    selector: _ -> [_ _]
    frame False {
      n330 = case shown="True" {
        selector: _ -> [_ _]
        tunnel: 0.5 ("Output") -> [_ w776]
        frame False {
          w771 = T9 0 items=["PercentOutput"=0, "Position"=1, "Velocity"=2, "Current"=3, "Follower"=5, "MotionProfile"=6, "MotionMagic"=7, "MotionProfileArc"=10, "Disabled"=15] ("Control Mode")
          n331 = call <vilib>:"CTRE_Phoenix_MotorControl_RefNumRegistryGet.vi"("refnum name"="abraco") -> ("error out"=w773:errorcluster, "PhoenixMotorControlDevRef"=w774:T3)  [unwired: 9 in]
          n332 = call <vilib>:"CTRE_Phoenix_MotorControl_Set.vi"("error in (no error)"=w773, "Output"=0.0, "Control Mode"=w771, "PhoenixMotorControlDevRef"=w774) -> ()  [unwired: 6 in, 2 out]
        }
        frame True {
          w777 = T9 0 items=["PercentOutput"=0, "Position"=1, "Velocity"=2, "Current"=3, "Follower"=5, "MotionProfile"=6, "MotionMagic"=7, "MotionProfileArc"=10, "Disabled"=15] ("Control Mode")
          n333 = Negate(x=w776) -> (-x=w775:dbl)
          n334 = call <vilib>:"CTRE_Phoenix_MotorControl_RefNumRegistryGet.vi"("refnum name"="abraco") -> ("error out"=w779:errorcluster, "PhoenixMotorControlDevRef"=w778:T3)  [unwired: 9 in]
          n335 = call <vilib>:"CTRE_Phoenix_MotorControl_Set.vi"("error in (no error)"=w779, "Output"=w775, "Control Mode"=w777, "PhoenixMotorControlDevRef"=w778) -> ()  [unwired: 6 in, 2 out]
        }
      }
    }
    frame True {
      w781 = T9 0 items=["PercentOutput"=0, "Position"=1, "Velocity"=2, "Current"=3, "Follower"=5, "MotionProfile"=6, "MotionMagic"=7, "MotionProfileArc"=10, "Disabled"=15] ("Control Mode")
      n336 = call <vilib>:"CTRE_Phoenix_MotorControl_RefNumRegistryGet.vi"("refnum name"="abraco") -> ("error out"=w783:errorcluster, "PhoenixMotorControlDevRef"=w784:T3)  [unwired: 9 in]
      n337 = call <vilib>:"CTRE_Phoenix_MotorControl_Set.vi"("error in (no error)"=w783, "Output"=0.5, "Control Mode"=w781, "PhoenixMotorControlDevRef"=w784) -> ()  [unwired: 6 in, 2 out]
    }
  }
  n338 = case shown="False" {
    selector: _ -> [_ _]
    frame False {
      n339 = case shown="True" {
        selector: _ -> [_ _]
        tunnel: 0.5 ("Output") -> [_ w793]
        frame False {
          w788 = T9 0 items=["PercentOutput"=0, "Position"=1, "Velocity"=2, "Current"=3, "Follower"=5, "MotionProfile"=6, "MotionMagic"=7, "MotionProfileArc"=10, "Disabled"=15] ("Control Mode")
          n340 = call <vilib>:"CTRE_Phoenix_MotorControl_RefNumRegistryGet.vi"("refnum name"="abraco") -> ("error out"=w790:errorcluster, "PhoenixMotorControlDevRef"=w791:T3)  [unwired: 9 in]
          n341 = call <vilib>:"CTRE_Phoenix_MotorControl_Set.vi"("error in (no error)"=w790, "Output"=0.0, "Control Mode"=w788, "PhoenixMotorControlDevRef"=w791) -> ()  [unwired: 6 in, 2 out]
        }
        frame True {
          w794 = T9 0 items=["PercentOutput"=0, "Position"=1, "Velocity"=2, "Current"=3, "Follower"=5, "MotionProfile"=6, "MotionMagic"=7, "MotionProfileArc"=10, "Disabled"=15] ("Control Mode")
          n342 = Negate(x=w793) -> (-x=w792:dbl)
          n343 = call <vilib>:"CTRE_Phoenix_MotorControl_RefNumRegistryGet.vi"("refnum name"="abraco") -> ("error out"=w796:errorcluster, "PhoenixMotorControlDevRef"=w795:T3)  [unwired: 9 in]
          n344 = call <vilib>:"CTRE_Phoenix_MotorControl_Set.vi"("error in (no error)"=w796, "Output"=w792, "Control Mode"=w794, "PhoenixMotorControlDevRef"=w795) -> ()  [unwired: 6 in, 2 out]
        }
      }
    }
    frame True {
      w798 = T9 0 items=["PercentOutput"=0, "Position"=1, "Velocity"=2, "Current"=3, "Follower"=5, "MotionProfile"=6, "MotionMagic"=7, "MotionProfileArc"=10, "Disabled"=15] ("Control Mode")
      n345 = call <vilib>:"CTRE_Phoenix_MotorControl_RefNumRegistryGet.vi"("refnum name"="abraco") -> ("error out"=w800:errorcluster, "PhoenixMotorControlDevRef"=w801:T3)  [unwired: 9 in]
      n346 = call <vilib>:"CTRE_Phoenix_MotorControl_Set.vi"("error in (no error)"=w800, "Output"=0.5, "Control Mode"=w798, "PhoenixMotorControlDevRef"=w801) -> ()  [unwired: 6 in, 2 out]
    }
  }
  n347 = call <vilib>:"WPI_JoystickRefNum Registry Get.vi"("refnum name"="Joystick 0") -> ("JoystickDevRef"=w62:T11)  [unwired: 1 in, 9 out]
  n348 = call <vilib>:"WPI_JoystickRefNum Registry Get.vi"("refnum name"="Joystick 0") -> ("error out"=w171:errorcluster, "JoystickDevRef"=w172:T11)  [unwired: 1 in, 8 out]
  n349 = call <vilib>:"WPI_JoystickRefNum Registry Get.vi"("refnum name"="Joystick 0") -> ("error out"=w152:errorcluster, "JoystickDevRef"=w151:T11)  [unwired: 1 in, 8 out]
  n350 = call <vilib>:"WPI_JoystickRefNum Registry Get.vi"("refnum name"="Joystick 0") -> ("JoystickDevRef"=w121:T11)  [unwired: 1 in, 9 out]
  n351 = Unbundle By Name("input cluster 2") -> ("Axes[1]"=w78:dbl, "Axes[2]"=w79:dbl, "Axes[3]"=w92:dbl)
  "Axes[1] 2" <- w78
  "Axes[2] 2" <- w79
  "Axes[3] 2" <- w92
  n352 = call <vilib>:"WPI_JoystickRefNum Registry Get.vi"("refnum name"="Joystick 0") -> ("JoystickDevRef"=w185:T11)  [unwired: 1 in, 9 out]
  n353 = call <vilib>:"WPI_JoystickGetValues.vi"("JoystickDevRef"=w55) -> ("POVs"=w51:i16[])  [unwired: 6 in, 4 out]
  n354 = call <vilib>:"WPI_JoystickGetValues.vi"("error in (no error)"=w171, "JoystickDevRef"=w172) -> ("Buttons"=w174:bool[])  [unwired: 5 in, 4 out]
  n355 = call <vilib>:"WPI_JoystickGetValues.vi"("error in (no error)"=w152, "JoystickDevRef"=w151) -> ("Buttons"=w149:bool[])  [unwired: 5 in, 4 out]
  n356 = call <vilib>:"WPI_JoystickGetValues.vi"("JoystickDevRef"=w62) -> ("POVs"=w58:i16[])  [unwired: 6 in, 4 out]
  n357 = Wait (ms)(milliseconds to wait=40) -> ()  [unwired: 1 out]
  n358 = call <vilib>:"WPI_JoystickGetValues.vi"("JoystickDevRef"=w121) -> ("Axes"=w119:dbl[])  [unwired: 6 in, 4 out]
  n359 = call <vilib>:"WPI_JoystickRefNum Registry Get.vi"("refnum name"="Joystick 0") -> ("JoystickDevRef"=w71:T11)  [unwired: 1 in, 9 out]
  n360 = call <vilib>:"WPI_JoystickGetValues.vi"("JoystickDevRef"=w185) -> ("Axes"=w183:dbl[])  [unwired: 6 in, 4 out]
  n361 = Array To Cluster(array=w174) -> (cluster=w162:T13)
  n362 = Array To Cluster(array=w149) -> (cluster=w161:T13)
  n363 = Array To Cluster(array=w51) -> (cluster=w50:T14)
  n364 = Array To Cluster(array=w58) -> (cluster=w57:T14)
  n365 = call <vilib>:"WPI_JoystickRefNum Registry Get.vi"("refnum name"="Joystick 0") -> ("JoystickDevRef"=w193:T11)  [unwired: 1 in, 9 out]
  n366 = Array To Cluster(array=w119) -> (cluster=w118:T1)
  n367 = call <vilib>:"WPI_JoystickGetValues.vi"("JoystickDevRef"=w71) -> ("Buttons"=w72:bool[])  [unwired: 6 in, 4 out]
  n368 = Unbundle By Name(w162) -> ("Buttons[4]"=w163:bool, "Buttons[5]"=w164:bool)
  "Buttons 11" <- w163
  "Buttons 10" <- w164
  n369 = Array To Cluster(array=w183) -> (cluster=w182:T1)
  n370 = Unbundle By Name(w161) -> ("Buttons[4]"=w160:bool, "Buttons[5]"=w159:bool)
  "Buttons 13" <- w160
  "Buttons 12" <- w159
  n371 = Unbundle By Name(w50) -> ("POVs[0]"=w49:i16)
  n372 = Unbundle By Name(w57) -> ("POVs[0]"=w56:i16)
  n373 = Negate(x=w79) -> (-x=w80:dbl)
  n374 = call <vilib>:"WPI_JoystickGetValues.vi"("JoystickDevRef"=w193) -> ("Axes"=w195:dbl[])  [unwired: 6 in, 4 out]
  n375 = Array To Cluster(array=w72) -> (cluster=w73:T10)
  n376 = Less?(x="x 2", y=0.0) -> (x < y?=w107:bool)
  n377 = local read "pwm_shot 2"() -> (w40:dbl)
  n378 = global read "GlobalVariables.vi" "Buttons_axes"() -> (w37:bool)
  n379 = call <vilib>:"WPI_RobotDriveRefNum Registry Get.vi"("refnum name"="Left and Right Motors") -> ("error out"=w199:errorcluster, "RobotDriveDevRef"=w198:T2)  [unwired: 9 in]
  n380 = Array To Cluster(array=w195) -> (cluster=w196:T1)
  n381 = Unbundle By Name(w118) -> ("Axes[1]"=w123:dbl, "Axes[2]"=w124:dbl, "Axes[3]"=w125:dbl, "Axes[4]"=w126:dbl)
  n382 = Add(x=w80, y=w92) -> (x+y=w94:dbl)
  n383 = Unbundle By Name(w73) -> ("Buttons[2]"=w77:bool, "Buttons[1]"=w76:bool, "Buttons[0]"=w74:bool, "Buttons[3]"=w75:bool)
  n384 = call <vilib>:"WPI_RobotDriveRefNum Registry Get.vi"("refnum name"="Left and Right Motors") -> ("error out"=w115:errorcluster, "RobotDriveDevRef"=w116:T2)  [unwired: 9 in]
  n385 = local write "Negar 2"(w107) -> ()
  n386 = Not Equal?(x=w49, y=-1.0) -> (x != y?=w52:bool)
  n387 = Absolute Value(x="x 2") -> (abs(x)=w109:dbl)
  n388 = Not Equal?(x=w56, y=-1.0) -> (x != y?=w59:bool)
  n389 = Unbundle By Name(w182) -> ("Axes[0]"=w186:dbl, "Axes[1]"=w187:dbl, "Axes[2]"=w189:dbl, "Axes[3]"=w190:dbl)
  n390 = call <vilib>:"WPI_RobotDriveRefNum Registry Get.vi"("refnum name"="Left and Right Motors") -> ("error out"=w179:errorcluster, "RobotDriveDevRef"=w180:T2)  [unwired: 9 in]
  n391 = global read "GlobalVariables.vi" "Aim_Lock"() -> (w38:bool)
  n392 = global read "GlobalVariables.vi" "Aim_Lock"() -> (w91:bool)
  n393 = Absolute Value(x=w40) -> (abs(x)=w41:dbl)
  n394 = call "Vi_por_infeite_deletar_depois.vi"("Numeric"=w94) -> ("Numeric 4"=w93:dbl)  [unwired: 8 in, 2 out]
  n395 = call "Vi_por_infeite_deletar_depois.vi"() -> ("Numeric 3"=w95:dbl)  [unwired: 9 in, 2 out]
  n396 = case shown="True" w52 {
    tunnel: w49 -> [_ w809]
    frame False {
      w804 = T9 0 items=["PercentOutput"=0, "Position"=1, "Velocity"=2, "Current"=3, "Follower"=5, "MotionProfile"=6, "MotionMagic"=7, "MotionProfileArc"=10, "Disabled"=15] ("Control Mode")
      n397 = call <vilib>:"CTRE_Phoenix_MotorControl_RefNumRegistryGet.vi"("refnum name"="elevador") -> ("error out"=w806:errorcluster, "PhoenixMotorControlDevRef"=w807:T3)  [unwired: 9 in]
      n398 = call <vilib>:"CTRE_Phoenix_MotorControl_Set.vi"("error in (no error)"=w806, "Output"=0.0, "Control Mode"=w804, "PhoenixMotorControlDevRef"=w807) -> ()  [unwired: 6 in, 2 out]
    }
    frame True {
      n399 = Equal?(x=w809, y=i16 0) -> (x = y?=w810:bool)
      n400 = case shown="False" w810 {
        tunnel: w809 -> [w813 _]
        tunnel: 0.4 ("Output") -> [w812 _]
        frame False {
          n401 = Equal?(x=w813, y=180.0) -> (x = y?=w815:bool)
          n402 = case shown="True" w815 {
            tunnel: w812 -> [_ w821]
            frame False {
              w818 = T9 0 items=["PercentOutput"=0, "Position"=1, "Velocity"=2, "Current"=3, "Follower"=5, "MotionProfile"=6, "MotionMagic"=7, "MotionProfileArc"=10, "Disabled"=15] ("Control Mode")
              n403 = call <vilib>:"CTRE_Phoenix_MotorControl_RefNumRegistryGet.vi"("refnum name"="elevador") -> ("error out"=w819:errorcluster, "PhoenixMotorControlDevRef"=w820:T3)  [unwired: 9 in]
              n404 = call <vilib>:"CTRE_Phoenix_MotorControl_Set.vi"("error in (no error)"=w819, "Output"=0.0, "Control Mode"=w818, "PhoenixMotorControlDevRef"=w820) -> ()  [unwired: 6 in, 2 out]
            }
            frame True {
              w824 = T9 0 items=["PercentOutput"=0, "Position"=1, "Velocity"=2, "Current"=3, "Follower"=5, "MotionProfile"=6, "MotionMagic"=7, "MotionProfileArc"=10, "Disabled"=15] ("Control Mode")
              # "reverses engine speed to down"
              n405 = Negate(x=w821) -> (-x=w822:dbl)
              n406 = call <vilib>:"CTRE_Phoenix_MotorControl_RefNumRegistryGet.vi"("refnum name"="elevador") -> ("error out"=w825:errorcluster, "PhoenixMotorControlDevRef"=w826:T3)  [unwired: 9 in]
              n407 = call <vilib>:"CTRE_Phoenix_MotorControl_Set.vi"("error in (no error)"=w825, "Output"=w822, "Control Mode"=w824, "PhoenixMotorControlDevRef"=w826) -> ()  [unwired: 6 in, 2 out]
            }
          }
        }
        frame True {
          n408 = global read "GlobalVariables.vi" "Disp_Valido"() -> (w827:dbl)
          n409 = Greater?(x=w827, y=10.0) -> (0:w830:bool)
          n410 = case shown="True" w830 {
            tunnel: 1.0 ("Output") -> [_ w836]
            frame False {
              w833 = T9 0 items=["PercentOutput"=0, "Position"=1, "Velocity"=2, "Current"=3, "Follower"=5, "MotionProfile"=6, "MotionMagic"=7, "MotionProfileArc"=10, "Disabled"=15] ("Control Mode")
              n411 = call <vilib>:"CTRE_Phoenix_MotorControl_RefNumRegistryGet.vi"("refnum name"="elevador") -> ("error out"=w834:errorcluster, "PhoenixMotorControlDevRef"=w835:T3)  [unwired: 9 in]
              n412 = call <vilib>:"CTRE_Phoenix_MotorControl_Set.vi"("error in (no error)"=w834, "Output"=0.0, "Control Mode"=w833, "PhoenixMotorControlDevRef"=w835) -> ()  [unwired: 6 in, 2 out]
            }
            frame True {
              w838 = T9 0 items=["PercentOutput"=0, "Position"=1, "Velocity"=2, "Current"=3, "Follower"=5, "MotionProfile"=6, "MotionMagic"=7, "MotionProfileArc"=10, "Disabled"=15] ("Control Mode")
              n413 = call <vilib>:"CTRE_Phoenix_MotorControl_RefNumRegistryGet.vi"("refnum name"="elevador") -> ("error out"=w839:errorcluster, "PhoenixMotorControlDevRef"=w840:T3)  [unwired: 9 in]
              n414 = call <vilib>:"CTRE_Phoenix_MotorControl_Set.vi"("error in (no error)"=w839, "Output"=w836, "Control Mode"=w838, "PhoenixMotorControlDevRef"=w840) -> ()  [unwired: 6 in, 2 out]
            }
          }
        }
      }
    }
  }
  n415 = Unbundle By Name(w196) -> ("Axes[1]"=w200:dbl, "Axes[2]"=w201:dbl)
  n416 = case shown="True" w59 {
    tunnel: w56 -> [_ w847]
    frame False {
      w842 = T9 0 items=["PercentOutput"=0, "Position"=1, "Velocity"=2, "Current"=3, "Follower"=5, "MotionProfile"=6, "MotionMagic"=7, "MotionProfileArc"=10, "Disabled"=15] ("Control Mode")
      n417 = call <vilib>:"CTRE_Phoenix_MotorControl_RefNumRegistryGet.vi"("refnum name"="elevador") -> ("error out"=w844:errorcluster, "PhoenixMotorControlDevRef"=w845:T3)  [unwired: 9 in]
      n418 = call <vilib>:"CTRE_Phoenix_MotorControl_Set.vi"("error in (no error)"=w844, "Output"=0.0, "Control Mode"=w842, "PhoenixMotorControlDevRef"=w845) -> ()  [unwired: 6 in, 2 out]
    }
    frame True {
      n419 = Equal?(x=w847, y=i16 0) -> (x = y?=w848:bool)
      n420 = case shown="True" w848 {
        tunnel: w847 -> [w851 _]
        tunnel: 0.4 ("Output") -> [w850 _]
        frame False {
          n421 = Equal?(x=w851, y=180.0) -> (x = y?=w853:bool)
          n422 = case shown="True" w853 {
            tunnel: w850 -> [_ w859]
            frame False {
              w856 = T9 0 items=["PercentOutput"=0, "Position"=1, "Velocity"=2, "Current"=3, "Follower"=5, "MotionProfile"=6, "MotionMagic"=7, "MotionProfileArc"=10, "Disabled"=15] ("Control Mode")
              n423 = call <vilib>:"CTRE_Phoenix_MotorControl_RefNumRegistryGet.vi"("refnum name"="elevador") -> ("error out"=w857:errorcluster, "PhoenixMotorControlDevRef"=w858:T3)  [unwired: 9 in]
              n424 = call <vilib>:"CTRE_Phoenix_MotorControl_Set.vi"("error in (no error)"=w857, "Output"=0.0, "Control Mode"=w856, "PhoenixMotorControlDevRef"=w858) -> ()  [unwired: 6 in, 2 out]
            }
            frame True {
              w862 = T9 0 items=["PercentOutput"=0, "Position"=1, "Velocity"=2, "Current"=3, "Follower"=5, "MotionProfile"=6, "MotionMagic"=7, "MotionProfileArc"=10, "Disabled"=15] ("Control Mode")
              n425 = Negate(x=w859) -> (-x=w860:dbl)
              n426 = call <vilib>:"CTRE_Phoenix_MotorControl_RefNumRegistryGet.vi"("refnum name"="elevador") -> ("error out"=w863:errorcluster, "PhoenixMotorControlDevRef"=w864:T3)  [unwired: 9 in]
              n427 = call <vilib>:"CTRE_Phoenix_MotorControl_Set.vi"("error in (no error)"=w863, "Output"=w860, "Control Mode"=w862, "PhoenixMotorControlDevRef"=w864) -> ()  [unwired: 6 in, 2 out]
            }
          }
        }
        frame True {
          n428 = local read "Disp_Valido"() -> (w867:dbl)
          n429 = Greater?(x=w867, y=10.0) -> (0:w868:bool)
          n430 = case shown="True" w868 {
            tunnel: 1.0 ("Output") -> [_ w874]
            frame False {
              w871 = T9 0 items=["PercentOutput"=0, "Position"=1, "Velocity"=2, "Current"=3, "Follower"=5, "MotionProfile"=6, "MotionMagic"=7, "MotionProfileArc"=10, "Disabled"=15] ("Control Mode")
              n431 = call <vilib>:"CTRE_Phoenix_MotorControl_RefNumRegistryGet.vi"("refnum name"="elevador") -> ("error out"=w872:errorcluster, "PhoenixMotorControlDevRef"=w873:T3)  [unwired: 9 in]
              n432 = call <vilib>:"CTRE_Phoenix_MotorControl_Set.vi"("error in (no error)"=w872, "Output"=0.0, "Control Mode"=w871, "PhoenixMotorControlDevRef"=w873) -> ()  [unwired: 6 in, 2 out]
            }
            frame True {
              w876 = T9 0 items=["PercentOutput"=0, "Position"=1, "Velocity"=2, "Current"=3, "Follower"=5, "MotionProfile"=6, "MotionMagic"=7, "MotionProfileArc"=10, "Disabled"=15] ("Control Mode")
              n433 = call <vilib>:"CTRE_Phoenix_MotorControl_RefNumRegistryGet.vi"("refnum name"="elevador") -> ("error out"=w877:errorcluster, "PhoenixMotorControlDevRef"=w878:T3)  [unwired: 9 in]
              n434 = call <vilib>:"CTRE_Phoenix_MotorControl_Set.vi"("error in (no error)"=w877, "Output"=w874, "Control Mode"=w876, "PhoenixMotorControlDevRef"=w878) -> ()  [unwired: 6 in, 2 out]
            }
          }
        }
      }
    }
  }
  n435 = global read "GlobalVariables.vi" "Aim_Lock"() -> (w43:bool)
  n436 = call "Vi_por_infeite_deletar_depois.vi"() -> ("Boolean"=w36:bool)  [unwired: 9 in, 2 out]
  n437 = Add(x=w125, y=w126) -> (x+y=w127:dbl)
  n438 = Multiply(x=w93, y=w95) -> (x*y=w83:dbl)
  n439 = Multiply(x=w78, y=w95) -> (x*y=w82:dbl)
  n440 = Add(x=w123, y=w124) -> (x+y=w122:dbl)
  n441 = Negate(x=w186) -> (-x=w188:dbl)
  n442 = Greater?(x=w41, y=0.1) -> (0:w42:bool)
  n443 = case shown="True" w91 {
    tunnel: w82 -> [w880 _]
    tunnel: w83 -> [w879 _]
    tunnel: [w880 w882] -> w84
    tunnel: [w879 w883] -> w85
    frame False {
    }
    frame True {
      # "The numbers inside the case \nare boundary variables and the \nVi's are the LimeLight calculations."
      # "global variable for \nthe location of the target."
      n444 = global read "GlobalVariables.vi" "ValidTarget"() -> (w881:bool)
      n445 = case shown="True" w881 {
        tunnel: [0.0 ("x+y") w890] -> w883
        tunnel: [0.0 ("x+y") w886] -> w882
        frame False {
        }
        frame True {
          (unwired) 0.35
          n446 = global read "GlobalVariables.vi" "Tx"() -> (w891:dbl)
          n447 = global read "GlobalVariables.vi" "Ty"() -> (w888:dbl)
          n448 = call "Vi_por_infeite_deletar_depois.vi"("Numeric 2"=w891, "Numeric"=0.6) -> ("Numeric 3"=w890:dbl)  [unwired: 7 in, 2 out]
          "L_Y 2" <- w890
          n449 = call "Vi_por_infeite_deletar_depois.vi"("Numeric 5"=0.3, "Numeric 2"=w888, "Numeric"=0.9) -> ("Numeric 4"=w886:dbl)  [unwired: 6 in, 2 out]
          "L_X 2" <- w886
        }
      }
    }
  }
  n450 = case shown="True" w38 {
    frame False {
      w894 = T9 0 items=["PercentOutput"=0, "Position"=1, "Velocity"=2, "Current"=3, "Follower"=5, "MotionProfile"=6, "MotionMagic"=7, "MotionProfileArc"=10, "Disabled"=15] ("Control Mode")
      n451 = call <vilib>:"CTRE_Phoenix_MotorControl_RefNumRegistryGet.vi"("refnum name"="disparador") -> ("error out"=w895:errorcluster, "PhoenixMotorControlDevRef"=w896:T3)  [unwired: 9 in]
      n452 = call <vilib>:"CTRE_Phoenix_MotorControl_Set.vi"("error in (no error)"=w895, "Output"=0.0, "Control Mode"=w894, "PhoenixMotorControlDevRef"=w896) -> ()  [unwired: 6 in, 2 out]
    }
    frame True {
      w903 = T9 0 items=["PercentOutput"=0, "Position"=1, "Velocity"=2, "Current"=3, "Follower"=5, "MotionProfile"=6, "MotionMagic"=7, "MotionProfileArc"=10, "Disabled"=15] ("Control Mode")
      # "Speed controlled via axis 2 and 3 (triggers L1 and R1)"
      n453 = call <vilib>:"WPI_JoystickRefNum Registry Get.vi"("refnum name"="Joystick 0") -> ("error out"=w910:errorcluster, "JoystickDevRef"=w909:T11)  [unwired: 1 in, 8 out]
      n454 = call <vilib>:"WPI_JoystickGetValues.vi"("error in (no error)"=w910, "JoystickDevRef"=w909) -> ("Axes"=w907:dbl[])  [unwired: 5 in, 4 out]
      n455 = Array To Cluster(array=w907) -> (cluster=w906:T19)
      n456 = Unbundle By Name(w906) -> ("Axes[2]"=w899:dbl, "Axes[3]"=w900:dbl)
      n457 = Negate(x=w900) -> (-x=w901:dbl)
      n458 = Add(x=w899, y=w901) -> (x+y=w898:dbl)
      "pwm_shot 2" <- w898
      n459 = call <vilib>:"CTRE_Phoenix_MotorControl_RefNumRegistryGet.vi"("refnum name"="disparador") -> ("error out"=w902:errorcluster, "PhoenixMotorControlDevRef"=w904:T3)  [unwired: 9 in]
      n460 = call <vilib>:"CTRE_Phoenix_MotorControl_Set.vi"("error in (no error)"=w902, "Output"=w898, "Control Mode"=w903, "PhoenixMotorControlDevRef"=w904) -> ()  [unwired: 6 in, 2 out]
    }
  }
  n461 = Add(x=w189, y=w190) -> (x+y=w192:dbl)
  n462 = Add(x=w188, y=w187) -> (x+y=w191:dbl)
  n463 = And(x=w42, y=w43) -> (x .and. y?=w44:bool)
  n464 = case shown="False" w77 {
    tunnel: w76 -> [w911 _]
    frame False {
      n465 = case shown="True" w911 {
        tunnel: 0.5 ("Output") -> [_ w919]
        frame False {
          w914 = T9 0 items=["PercentOutput"=0, "Position"=1, "Velocity"=2, "Current"=3, "Follower"=5, "MotionProfile"=6, "MotionMagic"=7, "MotionProfileArc"=10, "Disabled"=15] ("Control Mode")
          n466 = call <vilib>:"CTRE_Phoenix_MotorControl_RefNumRegistryGet.vi"("refnum name"="abraco") -> ("error out"=w916:errorcluster, "PhoenixMotorControlDevRef"=w917:T3)  [unwired: 9 in]
          n467 = call <vilib>:"CTRE_Phoenix_MotorControl_Set.vi"("error in (no error)"=w916, "Output"=0.0, "Control Mode"=w914, "PhoenixMotorControlDevRef"=w917) -> ()  [unwired: 6 in, 2 out]
        }
        frame True {
          w920 = T9 0 items=["PercentOutput"=0, "Position"=1, "Velocity"=2, "Current"=3, "Follower"=5, "MotionProfile"=6, "MotionMagic"=7, "MotionProfileArc"=10, "Disabled"=15] ("Control Mode")
          n468 = Negate(x=w919) -> (-x=w918:dbl)
          n469 = call <vilib>:"CTRE_Phoenix_MotorControl_RefNumRegistryGet.vi"("refnum name"="abraco") -> ("error out"=w922:errorcluster, "PhoenixMotorControlDevRef"=w921:T3)  [unwired: 9 in]
          n470 = call <vilib>:"CTRE_Phoenix_MotorControl_Set.vi"("error in (no error)"=w922, "Output"=w918, "Control Mode"=w920, "PhoenixMotorControlDevRef"=w921) -> ()  [unwired: 6 in, 2 out]
        }
      }
    }
    frame True {
      w924 = T9 0 items=["PercentOutput"=0, "Position"=1, "Velocity"=2, "Current"=3, "Follower"=5, "MotionProfile"=6, "MotionMagic"=7, "MotionProfileArc"=10, "Disabled"=15] ("Control Mode")
      n471 = call <vilib>:"CTRE_Phoenix_MotorControl_RefNumRegistryGet.vi"("refnum name"="abraco") -> ("error out"=w926:errorcluster, "PhoenixMotorControlDevRef"=w927:T3)  [unwired: 9 in]
      n472 = call <vilib>:"CTRE_Phoenix_MotorControl_Set.vi"("error in (no error)"=w926, "Output"=0.5, "Control Mode"=w924, "PhoenixMotorControlDevRef"=w927) -> ()  [unwired: 6 in, 2 out]
    }
  }
  n473 = case shown="True" w74 {
    selector: w74 -> [_ w943]
    tunnel: w75 -> [w929 _]
    frame False {
      # "Expulsar"
      n474 = case shown="False" w929 {
        tunnel: 0.9 -> [_ w937]
        frame False {
          w932 = T9 0 items=["PercentOutput"=0, "Position"=1, "Velocity"=2, "Current"=3, "Follower"=5, "MotionProfile"=6, "MotionMagic"=7, "MotionProfileArc"=10, "Disabled"=15] ("Control Mode")
          n475 = call <vilib>:"CTRE_Phoenix_MotorControl_RefNumRegistryGet.vi"("refnum name"="braco") -> ("error out"=w935:errorcluster, "PhoenixMotorControlDevRef"=w934:T3)  [unwired: 9 in]
          n476 = call <vilib>:"CTRE_Phoenix_MotorControl_Set.vi"("error in (no error)"=w935, "Output"=0.0, "Control Mode"=w932, "PhoenixMotorControlDevRef"=w934) -> ()  [unwired: 6 in, 2 out]
        }
        frame True {
          w939 = T9 0 items=["PercentOutput"=0, "Position"=1, "Velocity"=2, "Current"=3, "Follower"=5, "MotionProfile"=6, "MotionMagic"=7, "MotionProfileArc"=10, "Disabled"=15] ("Control Mode")
          n477 = Negate(x=w937) -> (-x=w936:dbl)
          n478 = call <vilib>:"CTRE_Phoenix_MotorControl_RefNumRegistryGet.vi"("refnum name"="braco") -> ("error out"=w940:errorcluster, "PhoenixMotorControlDevRef"=w941:T3)  [unwired: 9 in]
          n479 = call <vilib>:"CTRE_Phoenix_MotorControl_Set.vi"("error in (no error)"=w940, "Output"=w936, "Control Mode"=w939, "PhoenixMotorControlDevRef"=w941) -> ()  [unwired: 6 in, 2 out]
        }
      }
    }
    frame True {
      n480 = case shown="True" w943 {
        tunnel: 1.0 ("Output") -> [_ w951]
        frame False {
          w945 = T9 0 items=["PercentOutput"=0, "Position"=1, "Velocity"=2, "Current"=3, "Follower"=5, "MotionProfile"=6, "MotionMagic"=7, "MotionProfileArc"=10, "Disabled"=15] ("Control Mode")
          n481 = call <vilib>:"CTRE_Phoenix_MotorControl_RefNumRegistryGet.vi"("refnum name"="braco") -> ("error out"=w948:errorcluster, "PhoenixMotorControlDevRef"=w947:T3)  [unwired: 9 in]
          n482 = call <vilib>:"CTRE_Phoenix_MotorControl_Set.vi"("error in (no error)"=w948, "Output"=0.0, "Control Mode"=w945, "PhoenixMotorControlDevRef"=w947) -> ()  [unwired: 6 in, 2 out]
        }
        frame True {
          w950 = T9 0 items=["PercentOutput"=0, "Position"=1, "Velocity"=2, "Current"=3, "Follower"=5, "MotionProfile"=6, "MotionMagic"=7, "MotionProfileArc"=10, "Disabled"=15] ("Control Mode")
          n483 = call <vilib>:"CTRE_Phoenix_MotorControl_RefNumRegistryGet.vi"("refnum name"="braco") -> ("error out"=w952:errorcluster, "PhoenixMotorControlDevRef"=w953:T3)  [unwired: 9 in]
          n484 = call <vilib>:"CTRE_Phoenix_MotorControl_Set.vi"("error in (no error)"=w952, "Output"=w951, "Control Mode"=w950, "PhoenixMotorControlDevRef"=w953) -> ()  [unwired: 6 in, 2 out]
        }
      }
    }
  }
  n485 = case shown="True" w36 {
    frame False {
      w957 = T9 0 items=["PercentOutput"=0, "Position"=1, "Velocity"=2, "Current"=3, "Follower"=5, "MotionProfile"=6, "MotionMagic"=7, "MotionProfileArc"=10, "Disabled"=15] ("Control Mode")
      n486 = call <vilib>:"CTRE_Phoenix_MotorControl_RefNumRegistryGet.vi"("refnum name"="elevador_total") -> ("error out"=w956:errorcluster, "PhoenixMotorControlDevRef"=w955:T3)  [unwired: 9 in]
      n487 = call <vilib>:"CTRE_Phoenix_MotorControl_Set.vi"("error in (no error)"=w956, "Output"=0.0, "Control Mode"=w957, "PhoenixMotorControlDevRef"=w955) -> ()  [unwired: 6 in, 2 out]
    }
    frame True {
      w961 = T9 0 items=["PercentOutput"=0, "Position"=1, "Velocity"=2, "Current"=3, "Follower"=5, "MotionProfile"=6, "MotionMagic"=7, "MotionProfileArc"=10, "Disabled"=15] ("Control Mode")
      # "Axis that moves the robot elevator up or down."
      n488 = call <vilib>:"WPI_JoystickRefNum Registry Get.vi"("refnum name"="Joystick 0") -> ("JoystickDevRef"=w966:T11)  [unwired: 1 in, 9 out]
      n489 = call <vilib>:"WPI_JoystickGetValues.vi"("JoystickDevRef"=w966) -> ("Axes"=w964:dbl[])  [unwired: 6 in, 4 out]
      n490 = Array To Cluster(array=w964) -> (cluster=w965:T20)
      n491 = Unbundle By Name(w965) -> ("Axes[5]"=w959:dbl)
      n492 = call <vilib>:"CTRE_Phoenix_MotorControl_RefNumRegistryGet.vi"("refnum name"="elevador_total") -> ("error out"=w963:errorcluster, "PhoenixMotorControlDevRef"=w962:T3)  [unwired: 9 in]
      n493 = call <vilib>:"CTRE_Phoenix_MotorControl_Set.vi"("error in (no error)"=w963, "Output"=w959, "Control Mode"=w961, "PhoenixMotorControlDevRef"=w962) -> ()  [unwired: 6 in, 2 out]
    }
  }
  n494 = case shown="True" w91 {
    frame False {
      n495 = call-poly <vilib>:"NT Write Value.vi"("Numeric"=1.0, "Name"="/limelight/ledMode") -> ()  [unwired: 9 in, 1 out]
    }
    frame True {
      n496 = call-poly <vilib>:"NT Write Value.vi"("Numeric"=3.0, "Name"="/limelight/ledMode") -> ()  [unwired: 9 in, 1 out]
    }
  }
  n497 = call-poly <vilib>:"WPI_RobotDriveArcadeDrive.vi"("error in (no error)"=w199, "Y axis value"=w201, "X axis value"=w200, "RobotDriveDevRef"=w198) -> ()  [unwired: 5 in, 3 out]
  n498 = local read "Lime_Min 2"() -> (w103:dbl)
  n499 = feedback #12(0.0) -> (w47:dbl)
  n500 = case shown="True" w44 {
    tunnel: [0.0 w974] -> w45
    tunnel: w47 -> [_ w973]
    frame False {
    }
    frame True {
      n501 = Increment(x=w973) -> (x+1=w974:dbl)
    }
  }
  "Disp_Valido 2" <- w45
  n502 = feedback-in #12(w45) -> ()
  n503 = case shown="False" {
    selector: _ -> [_ w988]
    frame False {
      # "Expulsar"
      n504 = case shown="False" {
        selector: _ -> [_ _]
        tunnel: 0.9 -> [_ w982]
        frame False {
          w977 = T9 0 items=["PercentOutput"=0, "Position"=1, "Velocity"=2, "Current"=3, "Follower"=5, "MotionProfile"=6, "MotionMagic"=7, "MotionProfileArc"=10, "Disabled"=15] ("Control Mode")
          n505 = call <vilib>:"CTRE_Phoenix_MotorControl_RefNumRegistryGet.vi"("refnum name"="braco") -> ("error out"=w980:errorcluster, "PhoenixMotorControlDevRef"=w979:T3)  [unwired: 9 in]
          n506 = call <vilib>:"CTRE_Phoenix_MotorControl_Set.vi"("error in (no error)"=w980, "Output"=0.0, "Control Mode"=w977, "PhoenixMotorControlDevRef"=w979) -> ()  [unwired: 6 in, 2 out]
        }
        frame True {
          w984 = T9 0 items=["PercentOutput"=0, "Position"=1, "Velocity"=2, "Current"=3, "Follower"=5, "MotionProfile"=6, "MotionMagic"=7, "MotionProfileArc"=10, "Disabled"=15] ("Control Mode")
          n507 = Negate(x=w982) -> (-x=w981:dbl)
          n508 = call <vilib>:"CTRE_Phoenix_MotorControl_RefNumRegistryGet.vi"("refnum name"="braco") -> ("error out"=w985:errorcluster, "PhoenixMotorControlDevRef"=w986:T3)  [unwired: 9 in]
          n509 = call <vilib>:"CTRE_Phoenix_MotorControl_Set.vi"("error in (no error)"=w985, "Output"=w981, "Control Mode"=w984, "PhoenixMotorControlDevRef"=w986) -> ()  [unwired: 6 in, 2 out]
        }
      }
    }
    frame True {
      n510 = case shown="True" w988 {
        tunnel: 1.0 ("Output") -> [_ w996]
        frame False {
          w990 = T9 0 items=["PercentOutput"=0, "Position"=1, "Velocity"=2, "Current"=3, "Follower"=5, "MotionProfile"=6, "MotionMagic"=7, "MotionProfileArc"=10, "Disabled"=15] ("Control Mode")
          n511 = call <vilib>:"CTRE_Phoenix_MotorControl_RefNumRegistryGet.vi"("refnum name"="braco") -> ("error out"=w993:errorcluster, "PhoenixMotorControlDevRef"=w992:T3)  [unwired: 9 in]
          n512 = call <vilib>:"CTRE_Phoenix_MotorControl_Set.vi"("error in (no error)"=w993, "Output"=0.0, "Control Mode"=w990, "PhoenixMotorControlDevRef"=w992) -> ()  [unwired: 6 in, 2 out]
        }
        frame True {
          w995 = T9 0 items=["PercentOutput"=0, "Position"=1, "Velocity"=2, "Current"=3, "Follower"=5, "MotionProfile"=6, "MotionMagic"=7, "MotionProfileArc"=10, "Disabled"=15] ("Control Mode")
          n513 = call <vilib>:"CTRE_Phoenix_MotorControl_RefNumRegistryGet.vi"("refnum name"="braco") -> ("error out"=w997:errorcluster, "PhoenixMotorControlDevRef"=w998:T3)  [unwired: 9 in]
          n514 = call <vilib>:"CTRE_Phoenix_MotorControl_Set.vi"("error in (no error)"=w997, "Output"=w996, "Control Mode"=w995, "PhoenixMotorControlDevRef"=w998) -> ()  [unwired: 6 in, 2 out]
        }
      }
    }
  }
  n515 = case shown="False" {
    selector: _ -> [_ w1012]
    frame False {
      # "Expulsar"
      n516 = case shown="False" {
        selector: _ -> [_ _]
        tunnel: 0.9 -> [_ w1006]
        frame False {
          w1001 = T9 0 items=["PercentOutput"=0, "Position"=1, "Velocity"=2, "Current"=3, "Follower"=5, "MotionProfile"=6, "MotionMagic"=7, "MotionProfileArc"=10, "Disabled"=15] ("Control Mode")
          n517 = call <vilib>:"CTRE_Phoenix_MotorControl_RefNumRegistryGet.vi"("refnum name"="braco") -> ("error out"=w1004:errorcluster, "PhoenixMotorControlDevRef"=w1003:T3)  [unwired: 9 in]
          n518 = call <vilib>:"CTRE_Phoenix_MotorControl_Set.vi"("error in (no error)"=w1004, "Output"=0.0, "Control Mode"=w1001, "PhoenixMotorControlDevRef"=w1003) -> ()  [unwired: 6 in, 2 out]
        }
        frame True {
          w1008 = T9 0 items=["PercentOutput"=0, "Position"=1, "Velocity"=2, "Current"=3, "Follower"=5, "MotionProfile"=6, "MotionMagic"=7, "MotionProfileArc"=10, "Disabled"=15] ("Control Mode")
          n519 = Negate(x=w1006) -> (-x=w1005:dbl)
          n520 = call <vilib>:"CTRE_Phoenix_MotorControl_RefNumRegistryGet.vi"("refnum name"="braco") -> ("error out"=w1009:errorcluster, "PhoenixMotorControlDevRef"=w1010:T3)  [unwired: 9 in]
          n521 = call <vilib>:"CTRE_Phoenix_MotorControl_Set.vi"("error in (no error)"=w1009, "Output"=w1005, "Control Mode"=w1008, "PhoenixMotorControlDevRef"=w1010) -> ()  [unwired: 6 in, 2 out]
        }
      }
    }
    frame True {
      n522 = case shown="True" w1012 {
        tunnel: 1.0 ("Output") -> [_ w1020]
        frame False {
          w1014 = T9 0 items=["PercentOutput"=0, "Position"=1, "Velocity"=2, "Current"=3, "Follower"=5, "MotionProfile"=6, "MotionMagic"=7, "MotionProfileArc"=10, "Disabled"=15] ("Control Mode")
          n523 = call <vilib>:"CTRE_Phoenix_MotorControl_RefNumRegistryGet.vi"("refnum name"="braco") -> ("error out"=w1017:errorcluster, "PhoenixMotorControlDevRef"=w1016:T3)  [unwired: 9 in]
          n524 = call <vilib>:"CTRE_Phoenix_MotorControl_Set.vi"("error in (no error)"=w1017, "Output"=0.0, "Control Mode"=w1014, "PhoenixMotorControlDevRef"=w1016) -> ()  [unwired: 6 in, 2 out]
        }
        frame True {
          w1019 = T9 0 items=["PercentOutput"=0, "Position"=1, "Velocity"=2, "Current"=3, "Follower"=5, "MotionProfile"=6, "MotionMagic"=7, "MotionProfileArc"=10, "Disabled"=15] ("Control Mode")
          n525 = call <vilib>:"CTRE_Phoenix_MotorControl_RefNumRegistryGet.vi"("refnum name"="braco") -> ("error out"=w1021:errorcluster, "PhoenixMotorControlDevRef"=w1022:T3)  [unwired: 9 in]
          n526 = call <vilib>:"CTRE_Phoenix_MotorControl_Set.vi"("error in (no error)"=w1021, "Output"=w1020, "Control Mode"=w1019, "PhoenixMotorControlDevRef"=w1022) -> ()  [unwired: 6 in, 2 out]
        }
      }
    }
  }
  n527 = feedback #13(0.6 ("y")) -> (w176:dbl)
  n528 = feedback #14(0.6 ("y")) -> (w147:dbl)
  n529 = call-poly <vilib>:"WPI_RobotDriveArcadeDrive.vi"("error in (no error)"=w179, "Y axis value"=w192, "X axis value"=w191, "RobotDriveDevRef"=w180) -> ()  [unwired: 5 in, 3 out]
  n530 = feedback #15(FALSE) -> (w167:bool)
  n531 = feedback #16(FALSE) -> (w156:bool)
  n532 = Subtract(x="Mot_Max 2", y="Mot_Min 2") -> (x-y=w96:dbl)
  n533 = Subtract(x=w109, y=w103) -> (x-y=w97:dbl)
  n534 = feedback #17(FALSE) -> (w32:bool)
  n535 = call-poly <vilib>:"WPI_RobotDriveArcadeDrive.vi"("error in (no error)"=w115, "Y axis value"=w127, "X axis value"=w122, "RobotDriveDevRef"=w116) -> ()  [unwired: 5 in, 3 out]
  n536 = local read "Lime_Max 2"() -> (w104:dbl)
  n537 = feedback #18(FALSE) -> (w34:bool)
  n538 = case shown="False" w37 {
    tunnel: [w1026 w1034] -> w30
    tunnel: w32 -> [w1023 w1035]
    tunnel: w34 -> [w1025 w1033]
    tunnel: [w1024 w1032] -> w35
    frame False {
      n539 = case shown="False" w1025 {
        selector: w1025 -> [w1028 w1031]
        tunnel: [w1027 w1029] -> w1026
        tunnel: [w1028 w1030] -> w1024
        tunnel: w1023 -> [w1027 w1029]
        frame False {
        }
        frame True {
          n540 = Not(x=w1031) -> (.not. x?=w1030:bool)
        }
      }
    }
    frame True {
      n541 = case shown="False" w1033 {
        selector: w1033 -> [_ w1039]
        tunnel: w1035 -> [w1037 w1040]
        tunnel: [w1038 w1040] -> w1034
        tunnel: [TRUE w1039] -> w1032
        frame False {
          n542 = Not(x=w1037) -> (.not. x?=w1038:bool)
        }
        frame True {
        }
      }
    }
  }
  "OUT_PUT 2" <- w30
  n543 = feedback-in #17(w30) -> ()
  n544 = feedback-in #18(w35) -> ()
  n545 = feedback #19(FALSE) -> (w169:bool)
  n546 = case shown="True" w164 {
    tunnel: w163 -> [w1047 _]
    tunnel: [w1045 w1067] -> w178
    tunnel: w176 -> [w1046 w1068]
    tunnel: w167 -> [w1044 w1069]
    tunnel: [w1043 w1066] -> w168
    tunnel: w169 -> [w1042 w1065]
    tunnel: [w1041 w1065] -> w170
    frame False {
      n547 = case shown="True" w1047 {
        tunnel: w1046 -> [w1052 w1058]
        tunnel: [w1052 w1057] -> w1045
        tunnel: w1042 -> [w1051 w1056]
        tunnel: [w1050 w1055] -> w1041
        frame False {
          n548 = case shown="False" w1051 {
            selector: w1051 -> [w1053 _]
            tunnel: [w1053 FALSE] -> w1050
            frame False {
            }
            frame True {
            }
          }
        }
        frame True {
          n549 = case shown="False" w1056 {
            selector: w1056 -> [_ w1063]
            tunnel: w1058 -> [w1061 w1064]
            tunnel: [w1060 w1064] -> w1057
            tunnel: [TRUE w1063] -> w1055
            frame False {
              # "redutor de \nvelocidadde"
              n550 = Subtract(x=w1061, y=0.2) -> (x-y=w1060:dbl)
            }
            frame True {
            }
          }
        }
      }
      n551 = case shown="False" w1044 {
        selector: w1044 -> [w1048 _]
        tunnel: [w1048 FALSE] -> w1043
        frame False {
        }
        frame True {
        }
      }
    }
    frame True {
      n552 = case shown="False" w1069 {
        selector: w1069 -> [_ w1074]
        tunnel: w1068 -> [w1072 w1075]
        tunnel: [w1071 w1075] -> w1067
        tunnel: [TRUE w1074] -> w1066
        frame False {
          # "Increase \nspeed."
          n553 = Add(x=w1072, y=0.2) -> (x+y=w1071:dbl)
        }
        frame True {
        }
      }
    }
  }
  "Mutliple" <- w178
  n554 = feedback-in #15(w168) -> ()
  n555 = feedback-in #19(w170) -> ()
  n556 = feedback #20(FALSE) -> (w154:bool)
  n557 = case shown="False" w159 {
    tunnel: w160 -> [w1082 _]
    tunnel: [w1080 w1102] -> w145
    tunnel: w147 -> [w1081 w1103]
    tunnel: w156 -> [w1079 w1104]
    tunnel: [w1078 w1101] -> w155
    tunnel: w154 -> [w1077 w1100]
    tunnel: [w1076 w1100] -> w153
    frame False {
      n558 = case shown="True" w1082 {
        tunnel: w1081 -> [w1087 w1093]
        tunnel: [w1087 w1092] -> w1080
        tunnel: w1077 -> [w1086 w1091]
        tunnel: [w1085 w1090] -> w1076
        frame False {
          n559 = case shown="False" w1086 {
            selector: w1086 -> [w1088 _]
            tunnel: [w1088 FALSE] -> w1085
            frame False {
            }
            frame True {
            }
          }
        }
        frame True {
          n560 = case shown="False" w1091 {
            selector: w1091 -> [_ w1098]
            tunnel: w1093 -> [w1096 w1099]
            tunnel: [w1095 w1099] -> w1092
            tunnel: [TRUE w1098] -> w1090
            frame False {
              # "Speed \nreducer"
              n561 = Subtract(x=w1096, y=0.2) -> (x-y=w1095:dbl)
            }
            frame True {
            }
          }
        }
      }
      n562 = case shown="False" w1079 {
        selector: w1079 -> [w1083 _]
        tunnel: [w1083 FALSE] -> w1078
        frame False {
        }
        frame True {
        }
      }
    }
    frame True {
      n563 = case shown="False" w1104 {
        selector: w1104 -> [_ w1109]
        tunnel: w1103 -> [w1107 w1110]
        tunnel: [w1106 w1110] -> w1102
        tunnel: [TRUE w1109] -> w1101
        frame False {
          # "increase \nspeed."
          n564 = Add(x=w1107, y=0.2) -> (x+y=w1106:dbl)
        }
        frame True {
        }
      }
    }
  }
  "Mutliple" <- w145
  n565 = feedback-in #16(w155) -> ()
  n566 = feedback-in #20(w153) -> ()
  n567 = Multiply(x=w96, y=w97) -> (x*y=w98:dbl)
  n568 = Subtract(x=w104, y=w103) -> (x-y=w99:dbl)
  n569 = call "Vi_por_infeite_deletar_depois.vi"("Numeric"=w178) -> ("Numeric 3"=w177:dbl)  [unwired: 8 in, 2 out]
  "OUT 4" <- w177
  n570 = feedback-in #13(w177) -> ()
  n571 = call "Vi_por_infeite_deletar_depois.vi"("Numeric"=w145) -> ("Numeric 3"=w146:dbl)  [unwired: 8 in, 2 out]
  "OUT 5" <- w146
  n572 = feedback-in #14(w146) -> ()
  n573 = Divide(x=w98, y=w99) -> (x/y=w100:dbl)
  n574 = local read "Negar 2"() -> (w110:bool)
  n575 = Add(x=w100, y="Mot_Min 2") -> (x+y=w111:dbl)
  n576 = case shown="True" w110 {
    tunnel: w111 -> [w1111 w1113]
    tunnel: [w1111 w1112] -> w112
    frame False {
    }
    frame True {
      n577 = Negate(x=w1113) -> (-x=w1112:dbl)
    }
  }
  "x+y 2" <- w112
  n578 = call <vilib>:"WPI_RobotDriveRefNum Registry Get.vi"("refnum name"="Left and Right Motors") -> ("error out"=w89:errorcluster, "RobotDriveDevRef"=w87:T2)  [unwired: 9 in]
  n579 = call-poly <vilib>:"WPI_RobotDriveArcadeDrive.vi"("error in (no error)"=w89, "Y axis value"=w84, "X axis value"=w85, "RobotDriveDevRef"=w87) -> ("Motor Values"=→"Motor Values  2":dbl[], "RobotDriveDevRef"=→"RobotDriveDevRef 2":T2)  [unwired: 5 in, 1 out]
  "Lime_Max" <- 20.0 ("x")
  "Lime_Min" <- 0.3 ("x")
  "Negar" <- FALSE
  "Lime_Max 2" <- 20.0 ("x")
  "Lime_Min 2" <- 0.3 ("x")
  "Negar 2" <- FALSE
